vi "psp_supervision.vi"() -> ()   [LabVIEW 2020]
uses:
  archive.ctl
  sync_type_def.ctl
  HT_type-def.ctl
  HF_type_def.ctl
  vacuum_type_def.ctl
  modulator_type_def.ctl
  water_cooling_type_def.ctl
  all_magnets_type_def.ctl
  <resource>/objmgr/ni.var.rc
panel:
  in  "container refnum in":refnum<k21>="ni.var.psp://eureka/SUPERVISION"
  out "archive":T1={"sync"={"elyse/sync/NI6071E/delay"=1.5500000000000005, "elyse/sync/NI6071E/width"=1.0, "elyse/sync/frequency/delay"=10.0, "elyse/sync/frequency/width"=181000.0, "elyse/sync/WCM/delay"=2177.9, "elyse/sync/WCM/width"=10.0, "elyse/sync/modulator/delay"=2182.400000000002, "elyse/sync/modulator/width"=3.0, "elyse/sync/HF/delay"=2175.0, "elyse/sync/HF/width"=3.0, "elyse/sync/Faraday/delay"=5080.0, "elyse/sync/Faraday/width"=100.0, "elyse/sync/Oscilloscope/delay"=2175.0, "elyse/sync/Oscilloscope/width"=2.8, "elyse/sync/50Hz_20MHz/delay"=1.0, "elyse/sync/50Hz_20MHz/width"=5000.0, "elyse/sync/laser_HF/delay"=0.35, "elyse/sync/laser_HF/width"=0.35, "elyse/sync/IMAC/delay"=2176.0, "elyse/sync/IMAC/width"=100.0, "elyse/sync/laser/delay"=2008.3, "elyse/sync/laser/width"=10.0, "elyse/sync/oscilloscope1/delay"=2175.0, "elyse/sync/oscilloscope1/width"=10.0, "elyse/sync/oscilloscope2/delay"=2175.0, "elyse/sync/oscilloscope2/width"=100.0, "elyse/sync/detection1/delay"=500.0, "elyse/sync/detection1/width"=500.0, "elyse/sync/detection1/delay"=0.3, "elyse/sync/detection2/width"=10.0, "elyse/sync/machine/delay"=2175.0, "elyse/sync/machine/width"=100.0, "elyse/sync/n_selection"=4.0}, "HT"={"elyse/HT/voltage/set_value"=6.5, "elyse/HT/voltage/value"=1.5625e-08, "elyse/HT/current/value"=0.0, "elyse/preamplifier/set_value"=1.5625e-08, "elyse/preamplifier/value"=0.0}, "HF"={"elyse/HF/attenuator/value"=-0.01903046052094623, "elyse/HF/dephaser/value"=-18.585806237727724, "elyse/HF/dephaser/value_manuel"=-78.82860725035081, "elyse/HF/canon/value"=0.0, "elyse/HF/section/value"=-18.585806237727724}, "vacuum"={"elyse/vacuum/preparation_chamber/state"=TRUE, "elyse/vacuum/preparation_chamber/measurement"=0.0, "elyse/vacuum/HF/state"=TRUE, "elyse/vacuum/HF/measurement"=0.0, "elyse/vacuum/canon/state"=TRUE, "elyse/vacuum/canon/measurement"=0.0, "elyse/vacuum/section/state"=TRUE, "elyse/vacuum/section/measurement"=0.0, "elyse/vacuum/dipole1/state"=TRUE, "elyse/vacuum/dipole1/measurement"=0.0, "elyse/vacuum/screen1/state"=TRUE, "elyse/vacuum/screen1/measurement"=0.0, "elyse/vacuum/mirror/state"=TRUE, "elyse/vacuum/mirror/measurement"=0.0, "elyse/vacuum/tpg300_section/state"=TRUE, "elyse/vacuum/tpg300_section/measurement"=0.0, "elyse/vacuum/valves/cathode/state"=FALSE, "elyse/vacuum/valves/injection/state"=FALSE}, "modulator"={"elyse/modulator/focale1/current/value"=0.0, "elyse/modulator/focale2/current/value"=0.0, "elyse/modulator/focale3/current/value"=0.0, "elyse/modulator/LAR/voltage/value"=0.0, "elyse/modulator/line_end/current/value"=0.0, "elyse/modulator/thyratron/currents/power/value"=0.0, "elyse/modulator/thyratron_reservoir/current/value"=0.0, "elyse/modulator/paramagnetization/current/value"=0.0, "elyse/modulator/thyratron/voltages/heating/value"=0.0, "elyse/modulator/thyratron/currents/heating/value"=0.0, "elyse/modulator/klystron/currents/power/value"=0.0, "elyse/modulator/klystron/voltages/power/value"=0.0, "elyse/modulator/klystron/currents/heating/value"=0.0, "elyse/modulator/klystron/voltages/heating/value"=0.0}, "cooling"={"elyse/cooling/section/temperature/set_value"=28.0, "elyse/cooling/section/temperature/measurement"=27.96142578125, "elyse/cooling/canon/temperature/set_value"=20.2, "elyse/cooling/canon/temperature/measurement"=26.69921875}, "magnets"={"elyse/magnets/focale/set_value"=0.0, "elyse/magnets/focale/value"=0.0, "elyse/magnets/phase_HF_laser/set_value"=0.0, "elyse/magnets/phase_HF_laser/value"=0.0, "elyse/magnets/dipole1/set_value"=0.0, "elyse/magnets/dipole1/value"=0.0, "elyse/magnets/dipole2/set_value"=0.0, "elyse/magnets/dipole2/value"=0.0, "elyse/magnets/Cor_H1/set_value"=0.0, "elyse/magnets/Cor_H1/value"=0.0, "elyse/magnets/Cor_V1/set_value"=0.0, "elyse/magnets/Cor_V1/value"=0.0, "elyse/magnets/Cor_H2/set_value"=0.0, "elyse/magnets/Cor_H2/value"=0.0, "elyse/magnets/Cor_V2/set_value"=0.0, "elyse/magnets/Cor_V2/value"=0.0, "elyse/magnets/Cor_H3/set_value"=0.0, "elyse/magnets/Cor_H3/value"=0.0, "elyse/magnets/Cor_V3/set_value"=-5.0, "elyse/magnets/Cor_V3/value"=0.0, "elyse/magnets/Cor_H4/set_value"=0.0, "elyse/magnets/Cor_H4/value"=0.0, "elyse/magnets/Cor_V4/set_value"=0.0, "elyse/magnets/Cor_V4/value"=0.0, "elyse/magnets/Cor_H5/set_value"=0.0, "elyse/magnets/Cor_H5/value"=0.0, "elyse/magnets/Cor_V5/set_value"=0.0, "elyse/magnets/Cor_V5/value"=0.0, "elyse/magnets/triplet1-1/set_value"=0.0, "elyse/magnets/triplet1-1/value"=0.0, "elyse/magnets/triplet1-2/set_value"=0.0, "elyse/magnets/triplet1-2/value"=0.0, "elyse/magnets/triplet2-1/set_value"=0.0, "elyse/magnets/triplet2-1/value"=0.0, "elyse/magnets/triplet2-2/set_value"=0.0, "elyse/magnets/triplet2-2/value"=0.0, "elyse/magnets/qudrupole1/set_value"=0.0, "elyse/magnets/qudrupole1/value"=0.0, "elyse/magnets/qudrupole2/set_value"=0.0, "elyse/magnets/qudrupole2/value"=0.0}, "time"={"elyse/timestamp"=0.0}}
  in  "Stop":bool
  out "Refnum SVE":refnum<k21>[](array[refnum])
  out "error out":errorcluster
  in  "tab":enum32{"  Variables"}(tab)
  in  "Onglet VAR PAR":T9(tab)=enum."C6/9 NI6703"
  out "DPS":T10
  out "EPS":T11
  out "DPC":T12
  out "EPC":T13
  out "C1NI6071E":T14 caption="Cluster 3" {"63 ACH63 b100 Libre ?" format="%.3f"; "62 ACH62 b98 Libre ?" format="%.3f"; "61 ACH61 b96 Libre ?" format="%.3f"; "60 ACH60 b94 Libre ?" format="%.3f"; "59 ACH59 b92 Libre ?" format="%.3f"; "58 ACH58 b90 Libre ?" format="%.3f"; "57 ACH57 b88 Libre ?" format="%.3f"; "56 ACH56 b86 Libre ?" format="%.3f"; "55 ACH55 b99 Libre ?" format="%.3f"; "54 ACH54 b97 Libre ?" format="%.3f"; "53 ACH53 b95 Libre ?" format="%.3f"; "52 ACH52 b93 Libre ?" format="%.3f"; "51 ACH51 b91 Libre ?" format="%.3f"; "50 ACH50 b89 Libre ?" format="%.3f"; "49 ACH49 b87 Libre ?" format="%.3f"; "48 ACH48 b85 Réservé" format="%.3f"; "47 ACH47 b84 Réservé" format="%.3f"; "46 ACH46 b82 Réservé" format="%.3f"; "45 ACH45 b80 Mesure phase HF1" format="%.3f"; "44 ACH44 b78 Mesure Atténuateur" format="%.3f"; "43 ACH43 b74 Réservé" format="%.3f"; "42 ACH42 b72 Mes champ Dipôle 2" format="%.3f"; "41 ACH41 b70 Mes H5" format="%.3f"; "40 ACH40 b68 Mes I correcte Dipôle 21 (H4)" format="%.3f"; "39 ACH39 b83 Réservé" format="%.3f"; "38 ACH38 b81 Mesure phase HF2" format="%.3f"; "37 ACH37 b79 Mes position Déphaseur ajust" format="%.3f"; "36 ACH36 b77 Mes position Déphaseur" format="%.3f"; "35 ACH35 b73 Mes champ Dipôle 2" format="%.3f"; "34 ACH34 b71 Mes I Guidage V5" format="%.3f"; "33 ACH33 b69 Mes I Guidage V4" format="%.3f"; "32 ACH32 b67 Mes I Guidage V3" format="%.3f"; "31 ACH31 b66 Mes I correcte Dipôle 1 (H3)" format="%.3f"; "30 ACH30 b64 Mes I Guidage H2" format="%.3f"; "29 ACH29 b62 Mes I Guidage H1" format="%.3f"; "28 ACH28 b60 Mes I Dipôle 1" format="%.3f"; "27 ACH27 b58 Mes I Quadripôle 2" format="%.3f"; "26 ACH26 b56 Réservé" format="%.3f"; "25 ACH25 b54 Mes I Triplet 2-1" format="%.3f"; "24 ACH24 b52 Mes I Triplet 1-2" format="%.3f"; "23 ACH23 b65 Mes I Guidage V2" format="%.3f"; "22 ACH22 b63 Mes I Guidage V1" format="%.3f"; "21 ACH21 b61 Mes I Dipôle 2" format="%.3f"; "20 ACH20 b59 Mes I Solénoïde" format="%.3f"; "19 ACH19 b57 Mes I Quadripôle 1" format="%.3f"; "18 ACH18 b55 Mes I Triplet 2-2" format="%.3f"; "17 ACH17 b53 Réservé" format="%.3f"; "16 ACH16 b51 Mes I Triplet 1-1" format="%.3f"; "15 ACH15 b18 Libre ?" format="%.3f"; "14 ACH14 b16 Libre ?" format="%.3f"; "13 ACH13 b14 Libre ?" format="%.3f"; "12 ACH12 b12 Mes Vide jauge canon" format="%.3f"; "11 ACH11 b10 Mes Vide DIP 1 (PIQ27 + 33)" format="%.3f"; "10 ACH10 b08 Mes Vide Section (PIQ 16)" format="%.3f"; "09 ACH09 b06 Mes Vide SAS guide HF" format="%.3f"; "08 ACH08 b04 Mes température Section" format="%.3f"; "07 ACH07 b17 Libre ?" format="%.3f"; "06 ACH06 b15 Libre ?" format="%.3f"; "05 ACH05 b13 Libre ?" format="%.3f"; "04 ACH04 b11 Mes Vide Ecran 1 (PIQ 53-63)" format="%.3f"; "03 ACH03 b09 Mes Vide Miroir (PIQ 21)" format="%.3f"; "02 ACH02 b07 Mes Vide Canon (PIQ 12)" format="%.3f"; "01 ACH01 b05 Mes Vide Chambre de préparation" format="%.3f"; "00 ACH00 b03 Mes température Canon" format="%.3f"}
  out "C2NI6071E":T15 caption="Cluster 3" {"63 ACH63 b100 Libre ?" format="%.3f"; "62 ACH62 b98 Libre ?" format="%.3f"; "61 ACH61 b96 Libre ?" format="%.3f"; "60 ACH60 b94 Libre ?" format="%.3f"; "59 ACH59 b92 Libre ?" format="%.3f"; "58 ACH58 b90 Libre ?" format="%.3f"; "57 ACH57 b88 Libre ?" format="%.3f"; "56 ACH56 b86 Signal laser 1" format="%.3f"; "55 ACH55 b99 Libre ?" format="%.3f"; "54 ACH54 b97 Libre ?" format="%.3f"; "53 ACH53 b95 Libre ?" format="%.3f"; "52 ACH52 b93 Libre ?" format="%.3f"; "51 ACH51 b91 Libre ?" format="%.3f"; "50 ACH50 b89 Libre ?" format="%.3f"; "49 ACH49 b87 Signal laser 2" format="%.3f"; "48 ACH48 b85 Mes position Miroir Y" format="%.3f"; "47 ACH47 b84 Mes position Miroir X" format="%.3f"; "46 ACH46 b82 Mes I obcs Faraday 3" format="%.3f"; "45 ACH45 b80 Mes I obcs Faraday 1" format="%.3f"; "44 ACH44 b78 Mes position Ecran 2" format="%.3f"; "43 ACH43 b74 Mes Fente V position mors B" format="%.3f"; "42 ACH42 b72 Mes Fente H position mors G" format="%.3f"; "41 ACH41 b70 Mes WCM 5" format="%.3f"; "40 ACH40 b68 Mes WCM 3" format="%.3f"; "39 ACH39 b83 Libre ?" format="%.3f"; "38 ACH38 b81 Mes I obcs Faraday 2" format="%.3f"; "37 ACH37 b79 Mes position Ecran 3" format="%.3f"; "36 ACH36 b77 Mes position Ecran 1" format="%.3f"; "35 ACH35 b73 Mes Fente V position mors H" format="%.3f"; "34 ACH34 b71 Mes Fente H position mors D" format="%.3f"; "33 ACH33 b69 Mes WCM 4" format="%.3f"; "32 ACH32 b67 Mes WCM 2D" format="%.3f"; "31 ACH31 b66 Mes WCM 2G" format="%.3f"; "30 ACH30 b64 Mes WCM 2H" format="%.3f"; "29 ACH29 b62 Mes WCM 1G" format="%.3f"; "28 ACH28 b60 Mes WCM 1H" format="%.3f"; "27 ACH27 b58 Mes I Faraday 2" format="%.3f"; "26 ACH26 b56 Mes HF directe Section" format="%.3f"; "25 ACH25 b54 Réservé" format="%.3f"; "24 ACH24 b52 Mes I Klystron" format="%.3f"; "23 ACH23 b65 Mes WCM 2B" format="%.3f"; "22 ACH22 b63 Mes WCM 1D" format="%.3f"; "21 ACH21 b61 Mes WCM 1B" format="%.3f"; "20 ACH20 b59 Mes I Faraday 3" format="%.3f"; "19 ACH19 b57 Mes I Faraday 1" format="%.3f"; "18 ACH18 b55 Mes HF directe Canon" format="%.3f"; "17 ACH17 b53 Mes V LAR" format="%.3f"; "16 ACH16 b51 Mes V Klystron" format="%.3f"; "15 ACH15 b18 Mes I alimentation HT" format="%.3f"; "14 ACH14 b16 Libre ?" format="%.3f"; "13 ACH13 b14 Mes I Focalisateur 2" format="%.3f"; "12 ACH12 b12 Mes I fin de Ligne" format="%.3f"; "11 ACH11 b10 Mes I Thyratron" format="%.3f"; "10 ACH10 b08 Mes I Réservoir Thyratron" format="%.3f"; "09 ACH09 b06 Mes I  Chauffage Klystron" format="%.3f"; "08 ACH08 b04 Mes I Chauffage Thyratron" format="%.3f"; "07 ACH07 b17 Mes V alimentation HT" format="%.3f"; "06 ACH06 b15 Mes I Focalisateur 3" format="%.3f"; "05 ACH05 b13 Mes I Focalisateur 1" format="%.3f"; "04 ACH04 b11 Mes I Prémagnétisation" format="%.3f"; "03 ACH03 b09 Réservé" format="%.3f"; "02 ACH02 b07 Mes I D'Qing" format="%.3f"; "01 ACH01 b05 Mes V Chauffage Klystron" format="%.3f"; "00 ACH00 b03 Mes V Chauffage Thyratron" format="%.3f"}
  out "C3_IN_DIO96":T16 caption="Cluster 3"
  out "C3_OUT_DIO96":T17 caption="Cluster 3"
  out "C4_IN_DIO96":T18 caption="Cluster 3"
  out "C4_OUT_DIO96":T19 caption="Cluster 3"
  out "C5_IN_DIO96":T20 caption="Cluster 3"
  out "C5_OUT_DIO96":T21 caption="Cluster 3"
  out "C6NI6703":T22 caption="Cluster 3" {"09 OUT09 b37 Cmd Guidage V5" format="%.3f"; "08 OUT08 b33 Réserve" format="%.3f"; "07 OUT07 b29 Cmd Guidage V4" format="%.3f"; "06 OUT06 b25 Cmd Guidage H4" format="%.3f"; "05 OUT05 b21 Cmd Guidage V3" format="%.3f"; "04 OUT04 b17 Cmd Guidage H3" format="%.3f"; "03 OUT03 b13 Cmd Guidage V2" format="%.3f"; "02 OUT02 b09 Cmd Guidage H2" format="%.3f"; "01 OUT01 b05 Cmd Guidage V1" format="%.3f"; "00 OUT00 b01 Cmd Guidage H1" format="%.3f"}
  out "C7NI6703":T23 caption="Cluster 3" {"09 OUT09 b37 Cmd I Dipôle 2" format="%.3f"; "08 OUT08 b33 Cmd I Dipôle 1" format="%.3f"; "07 OUT07 b29 Cmd I Quad 2" format="%.3f"; "06 OUT06 b25 Cmd I Quad 1" format="%.3f"; "05 OUT05 b21 Cmd I Solénoïde" format="%.3f"; "04 OUT04 b17 Cmd I Triplet 2-2" format="%.3f"; "03 OUT03 b13 Cmd I Triplet 2-1" format="%.3f"; "02 OUT02 b09 Réserve" format="%.3f"; "01 OUT01 b05 Cmd I Triplet 1-2" format="%.3f"; "00 OUT00 b01 Cmd I Triplet 1-1" format="%.3f"}
  out "C8NI6703":T24 caption="Cluster 3" {"09 OUT09 b37 Cmd position Miroir Y" format="%.3f"; "08 OUT08 b33 Cmd position Miroir X" format="%.3f"; "07 OUT07 b29 Réserve" format="%.3f"; "06 OUT06 b25 Cmd amplitude HF préampli" format="%.3f"; "05 OUT05 b21 Cmd déphasage HF/LASER" format="%.3f"; "04 OUT04 b17 Cmd Pos. Atténuateur" format="%.3f"; "03 OUT03 b13 Cmd Pos. Déphaseur" format="%.3f"; "02 OUT02 b09 Cmd Temp. Section" format="%.3f"; "01 OUT01 b05 Cmd Temp. Canon" format="%.3f"; "00 OUT00 b01 Réserve" format="%.3f"}
  out "C9NI6703":T25 caption="Cluster 3" {"09 OUT09 b37 Réserve" format="%.3f"; "08 OUT08 b33 Réserve" format="%.3f"; "07 OUT07 b29 Réserve" format="%.3f"; "06 OUT06 b25 Cmd position translateur Ecran 3" format="%.3f"; "05 OUT05 b21 Cmd position translateur Ecran 2" format="%.3f"; "04 OUT04 b17 Cmd position translateur Ecran 1" format="%.3f"; "03 OUT03 b13 Cmd position fente HD" format="%.3f"; "02 OUT02 b09 Cmd position fente HG" format="%.3f"; "01 OUT01 b05 Cmd DeQing" format="%.3f"; "00 OUT00 b01 Cmd alimentation HT" format="%.3f"}
  out "C1011NI6602":T26 caption="Cluster 3" {"N° du compteur" format="%.3f"; "31 OUT07 b16 C11 Largeur" format="%.3f"; "30 OUT07 b16 C11 Délais" format="%.3f"; "29 OUT06 b53 C11 Largeur" format="%.3f"; "28 OUT06 b53 C11 Délais" format="%.3f"; "27 OUT05 b23 C11 Largeur" format="%.3f"; "26 OUT05 b23 C11 Délais" format="%.3f"; "25 OUT04 b26 C11 Largeur" format="%.3f"; "24 OUT04 b26 C11 Délais" format="%.3f"; "23 OUT03 b29 C11 Largeur" format="%.3f"; "22 OUT03 b29 C11 Délais" format="%.3f"; "21 OUT02 b32 C11 Largeur" format="%.3f"; "20 OUT02 b32 C11 Délais" format="%.3f"; "19 OUT01 b09 C11 Largeur" format="%.3f"; "18 OUT01 b09 C11 Délais" format="%.3f"; "17 OUT00 b05 C11 Largeur" format="%.3f"; "16 OUT00 b05 C11 Délais" format="%.3f"; "15 OUT07 b16 C10 Largeur" format="%.3f"; "14 OUT07 b16 C10 Délais" format="%.3f"; "13 OUT06 b53 C10 Largeur" format="%.3f"; "12 OUT06 b53 C10 Délais" format="%.3f"; "11 OUT05 b23 C10 Largeur" format="%.3f"; "10 OUT05 b23 C10 Délais" format="%.3f"; "09 OUT04 b26 C10 Largeur" format="%.3f"; "08 OUT04 b26 C10 Délais" format="%.3f"; "07 OUT03 b29 C10 Largeur" format="%.3f"; "06 OUT03 b29 C10 Délais" format="%.3f"; "05 OUT02 b32 C10 Largeur" format="%.3f"; "04 OUT02 b32 C10 Délais" format="%.3f"; "03 OUT01 b09 C10 Largeur" format="%.3f"; "02 OUT01 b09 C10 Délais" format="%.3f"; "01 OUT00 b05 C10 Largeur" format="%.3f"; "00 OUT00 b05 C10 Délais" format="%.3f"}
  out "C12NI1409":string
  out "VDM-S":T27 caption="Cluster 3"
  out "VDM-A":T28 caption="Cluster 3"
  out "VDD":T27 caption="Cluster 3"
  out "VAM-S":T29 caption="Cluster 3" {"63" format="%.4g"; "62" format="%.4g"; "61" format="%.4g"; "60" format="%.4g"; "59" format="%.4g"; "58" format="%.4g"; "57" format="%.4g"; "56" format="%.4g"; "55" format="%.4g"; "54" format="%.4g"; "53" format="%.4g"; "52" format="%.4g"; "51" format="%.4g"; "50" format="%.4g"; "49" format="%.4g"; "48" format="%.4g"; "47" format="%.4g"; "46" format="%.4g"; "45" format="%.4g"; "44" format="%.4g"; "43" format="%.4g"; "42" format="%.4g"; "41" format="%.4g"; "40" format="%.4g"; "39" format="%.4g"; "38" format="%.4g"; "37" format="%.4g"; "36" format="%.4g"; "35" format="%.4g"; "34" format="%.4g"; "33" format="%.4g"; "32" format="%.4g"; "31" format="%.4g"; "30" format="%.4g"; "29" format="%.4g"; "28" format="%.4g"; "27" format="%.4g"; "26" format="%.4g"; "25" format="%.4g"; "24" format="%.4g"; "23" format="%.4g"; "22" format="%.4g"; "21" format="%.4g"; "20" format="%.4g"; "19" format="%.4g"; "18" format="%.4g"; "17" format="%.4g"; "16" format="%.4g"; "15" format="%.4g"; "14" format="%.4g"; "13" format="%.4g"; "12" format="%.4g"; "11" format="%.4g"; "10" format="%.4g"; "09" format="%.4g"; "08" format="%.4g"; "07" format="%.4g"; "06" format="%.4g"; "05" format="%.4g"; "04" format="%.4g"; "03" format="%.4g"; "02 SUP Evenement" format="%.4g"; "01 SUP Variables" format="%.4g"; "00 SUP Vidéo" format="%.4g"}
  out "VAM-A":T30 caption="Cluster 3" {"63 B_NI6220" format="%.4g"; "62" format="%.4g"; "61" format="%.4g"; "60" format="%.4g"; "59" format="%.4g"; "58" format="%.4g"; "57" format="%.4g"; "56" format="%.4g"; "55" format="%.4g"; "54" format="%.4g"; "53" format="%.4g"; "52" format="%.4g"; "51" format="%.4g"; "50" format="%.4g"; "49" format="%.4g"; "48" format="%.4g"; "47" format="%.4g"; "46" format="%.4g"; "45" format="%.4g"; "44" format="%.4g"; "43" format="%.4g"; "42" format="%.4g"; "41" format="%.4g"; "40" format="%.4g"; "39 WCM2DMin" format="%.4g"; "38 WCM2GMin" format="%.4g"; "37 WCM2BMin" format="%.4g"; "36 WCM2HMin" format="%.4g"; "35 WCM2DMax" format="%.4g"; "34 WCM2GMax" format="%.4g"; "33 WCM2BMax" format="%.4g"; "32 WCM2HMax" format="%.4g"; "31" format="%.4g"; "30" format="%.4g"; "29" format="%.4g"; "28" format="%.4g"; "27" format="%.4g"; "26" format="%.4g"; "25" format="%.4g"; "24" format="%.4g"; "23" format="%.4g"; "22" format="%.4g"; "21" format="%.4g"; "20 ACQ Vide TPG300 PIQ63" format="%.4g"; "19 ACQ Libre" format="%.5g"; "18 ACQ Libre" format="%.5g"; "17 ACQ Vide Ecran PIQ53/63" format="%.5g"; "16 ACQ Vide Dip PIQ27/33" format="%.5g"; "15 ACQ Vide Miroir PIQ21" format="%.5g"; "14 ACQ Vide Section PIQ16" format="%.5g"; "13 ACQ Vide Canon PIQ12" format="%.5g"; "12 ACQ Vide PI Guide HF" format="%.5f"; "11 ACQ Vide Chambre" format="%.4g"; "10 ACQ Vide Section" format="%.4g"; "09" format="%.4g"; "08" format="%.4g"; "07" format="%.4g"; "06" format="%.4g"; "05" format="%.4g"; "04" format="%.4g"; "03" format="%.4g"; "02 ACQ Evénement" format="%.4g"; "01 ACQ Variables" format="%.4g"; "00 ACQ Auxiliare" format="%.4g"}
  out "VAD":T31 caption="Cluster 3" {"63" format="%.4g"; "62" format="%.4g"; "61" format="%.4g"; "60" format="%.4g"; "59" format="%.4g"; "58" format="%.4g"; "57" format="%.4g"; "56" format="%.4g"; "55" format="%.4g"; "54" format="%.4g"; "53" format="%.4g"; "52" format="%.4g"; "51" format="%.4g"; "50" format="%.4g"; "49" format="%.4g"; "48" format="%.4g"; "47" format="%.4g"; "46" format="%.4g"; "45" format="%.4g"; "44" format="%.4g"; "43" format="%.4g"; "42" format="%.4g"; "41" format="%.4g"; "40" format="%.4g"; "39" format="%.4g"; "38" format="%.4g"; "37" format="%.4g"; "36" format="%.4g"; "35" format="%.4g"; "34" format="%.4g"; "33" format="%.4g"; "32" format="%.4g"; "31" format="%.4g"; "30" format="%.4g"; "29" format="%.4g"; "28" format="%.4g"; "27" format="%.4g"; "26" format="%.4g"; "25" format="%.4g"; "24" format="%.4g"; "23" format="%.4g"; "22" format="%.4g"; "21" format="%.4g"; "20" format="%.4g"; "19" format="%.4g"; "18" format="%.4g"; "17" format="%.4g"; "16" format="%.4g"; "15" format="%.4g"; "14" format="%.4g"; "13" format="%.4g"; "12" format="%.4g"; "11" format="%.4g"; "10" format="%.4g"; "09" format="%.4g"; "08" format="%.4g"; "07" format="%.4g"; "06" format="%.4g"; "05" format="%.4g"; "04" format="%.4g"; "03" format="%.4g"; "02" format="%.4g"; "01" format="%.4g"; "00" format="%.4g"}
  out "VTL":string[](array[string])
  out "VTS":string[](array[string])
  out "VTA":string[](array[string])
  # "Légende:\n\nLes Procédure simples sont des actions uniques sur un éléments ou groupe d'éléments.\nSelon les élements mis en oeuvre l'état OK de fin de procédure dépend de la remontée ou non de paramêtres de contrôle.\n\nLes Procédures combinées mettent en oeuvre une suites de procédures simples et correspondent à un état précis d'Elyse:\n(TIR - PRETIR-VEILLE - ARRET)\n\nSDC: Salle De Contrôle.\nX: Correspond à une demande de l'utilisateur depuis la SDC ou d'un pilotage distant.\nED: En Défaut.\nI: Etats transitoire (ex: entre TIR et Veille).\n1 2 3 4: correspond aux étapes intermédiaires de démarrage du modulateur.\nReset: Signifie une remise à zéro des défauts ce qui permet de passer à l'étape suivante.\nOK: Correspond à un une fin de procédure normale sans défaut.\nX EC: Correspond à un flag indiquant une demande de procédure combinée en cours.\nDPS: Cluster de Demande de Prcédure Simples (Read PC-ACQ / Write PC-SUP)\nEPS: Cluster d'Etats des Procédures Simples (Write PC-ACQ / Read PC-SUP)\nDPC: Cluster de Demande de Procédure Combinées (Read PC-ACQ / Write PC-SUP)\nEPC: Cluster d'états des Procédures Combinées (Write PC-ACQ / Read PC-SUP)"
  # "Cluster d'entrée des 64 voies analogiques de la carte C1 PCI 6071E"
  # "Cluster d'entrée des 64 voies analogiques de la carte C2 PCI 6071E"
  # "Cluster d'entrée des 56 voies numériques de la carte C3 DIO96"
  # "Cluster de sortie des 40 voies \nnumériques de la carte C3 DIO96"
  # "Cluster d'entrée des 64 voies numériques de la carte C4 DIO96"
  # "Cluster de sortie des 32 voies numériques \nde la carte C4 DIO96"
  # "Cluster d'entrée des 56 voies numériques de la carte C5 DIO96"
  # "Cluster de sortie des 40 voies numériques\nde la carte C5 DIO96"
  # "Cluster de sortie des 9 voies analogiques des 4 cartes C6,C7,C8,C9 PCI6703"
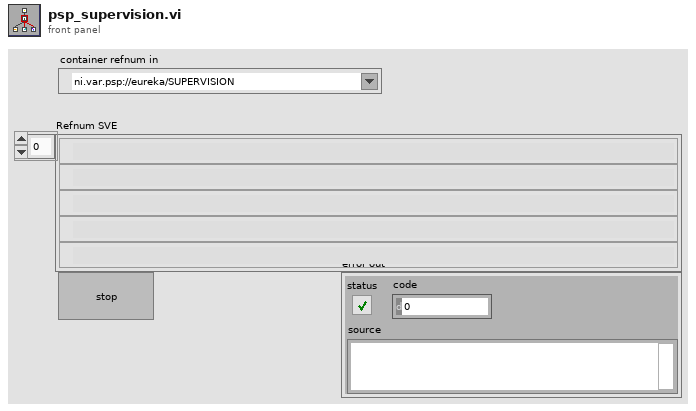
[diagram p1: front panel]
types:
  T1 = typedef "archive.ctl" = cluster{"sync":T2, "HT":T3, "HF":T4, "vacuum":T5, "modulator":T6, "cooling":T7, "magnets":T8, "time":cluster{"elyse/timestamp":dbl}}
  T2 = typedef "sync_type_def.ctl" = cluster{"elyse/sync/NI6071E/delay":dbl, "elyse/sync/NI6071E/width":dbl, "elyse/sync/frequency/delay":dbl, "elyse/sync/frequency/width":dbl, "elyse/sync/WCM/delay":dbl, "elyse/sync/WCM/width":dbl, "elyse/sync/modulator/delay":dbl, "elyse/sync/modulator/width":dbl, "elyse/sync/HF/delay":dbl, "elyse/sync/HF/width":dbl, "elyse/sync/Faraday/delay":dbl, "elyse/sync/Faraday/width":dbl, "elyse/sync/Oscilloscope/delay":dbl, "elyse/sync/Oscilloscope/width":dbl, "elyse/sync/50Hz_20MHz/delay":dbl, "elyse/sync/50Hz_20MHz/width":dbl, "elyse/sync/laser_HF/delay":dbl, "elyse/sync/laser_HF/width":dbl, "elyse/sync/IMAC/delay":dbl, "elyse/sync/IMAC/width":dbl, "elyse/sync/laser/delay":dbl, "elyse/sync/laser/width":dbl, "elyse/sync/oscilloscope1/delay":dbl, "elyse/sync/oscilloscope1/width":dbl, "elyse/sync/oscilloscope2/delay":dbl, "elyse/sync/oscilloscope2/width":dbl, "elyse/sync/detection1/delay":dbl, "elyse/sync/detection1/width":dbl, "elyse/sync/detection1/delay":dbl, "elyse/sync/detection2/width":dbl, "elyse/sync/machine/delay":dbl, "elyse/sync/machine/width":dbl, "elyse/sync/n_selection":dbl}
  T3 = typedef "HT_type-def.ctl" = cluster{"elyse/HT/voltage/set_value":dbl, "elyse/HT/voltage/value":dbl, "elyse/HT/current/value":dbl, "elyse/preamplifier/set_value":dbl, "elyse/preamplifier/value":dbl}
  T4 = typedef "HF_type_def.ctl" = cluster{"elyse/HF/attenuator/value":dbl, "elyse/HF/dephaser/value":dbl, "elyse/HF/dephaser/value_manuel":dbl, "elyse/HF/canon/value":dbl, "elyse/HF/section/value":dbl}
  T5 = typedef "vacuum_type_def.ctl" = cluster{"elyse/vacuum/preparation_chamber/state":bool, "elyse/vacuum/preparation_chamber/measurement":dbl, "elyse/vacuum/HF/state":bool, "elyse/vacuum/HF/measurement":dbl, "elyse/vacuum/canon/state":bool, "elyse/vacuum/canon/measurement":dbl, "elyse/vacuum/section/state":bool, "elyse/vacuum/section/measurement":dbl, "elyse/vacuum/dipole1/state":bool, "elyse/vacuum/dipole1/measurement":dbl, "elyse/vacuum/screen1/state":bool, "elyse/vacuum/screen1/measurement":dbl, "elyse/vacuum/mirror/state":bool, "elyse/vacuum/mirror/measurement":dbl, "elyse/vacuum/tpg300_section/state":bool, "elyse/vacuum/tpg300_section/measurement":dbl, "elyse/vacuum/valves/cathode/state":bool, "elyse/vacuum/valves/injection/state":bool}
  T6 = typedef "modulator_type_def.ctl" = cluster{"elyse/modulator/focale1/current/value":dbl, "elyse/modulator/focale2/current/value":dbl, "elyse/modulator/focale3/current/value":dbl, "elyse/modulator/LAR/voltage/value":dbl, "elyse/modulator/line_end/current/value":dbl, "elyse/modulator/thyratron/currents/power/value":dbl, "elyse/modulator/thyratron_reservoir/current/value":dbl, "elyse/modulator/paramagnetization/current/value":dbl, "elyse/modulator/thyratron/voltages/heating/value":dbl, "elyse/modulator/thyratron/currents/heating/value":dbl, "elyse/modulator/klystron/currents/power/value":dbl, "elyse/modulator/klystron/voltages/power/value":dbl, "elyse/modulator/klystron/currents/heating/value":dbl, "elyse/modulator/klystron/voltages/heating/value":dbl}
  T7 = typedef "water_cooling_type_def.ctl" = cluster{"elyse/cooling/section/temperature/set_value":dbl, "elyse/cooling/section/temperature/measurement":dbl, "elyse/cooling/canon/temperature/set_value":dbl, "elyse/cooling/canon/temperature/measurement":dbl}
  T8 = typedef "all_magnets_type_def.ctl" = cluster{"elyse/magnets/focale/set_value":dbl, "elyse/magnets/focale/value":dbl, "elyse/magnets/phase_HF_laser/set_value":dbl, "elyse/magnets/phase_HF_laser/value":dbl, "elyse/magnets/dipole1/set_value":dbl, "elyse/magnets/dipole1/value":dbl, "elyse/magnets/dipole2/set_value":dbl, "elyse/magnets/dipole2/value":dbl, "elyse/magnets/Cor_H1/set_value":dbl, "elyse/magnets/Cor_H1/value":dbl, "elyse/magnets/Cor_V1/set_value":dbl, "elyse/magnets/Cor_V1/value":dbl, "elyse/magnets/Cor_H2/set_value":dbl, "elyse/magnets/Cor_H2/value":dbl, "elyse/magnets/Cor_V2/set_value":dbl, "elyse/magnets/Cor_V2/value":dbl, "elyse/magnets/Cor_H3/set_value":dbl, "elyse/magnets/Cor_H3/value":dbl, "elyse/magnets/Cor_V3/set_value":dbl, "elyse/magnets/Cor_V3/value":dbl, "elyse/magnets/Cor_H4/set_value":dbl, "elyse/magnets/Cor_H4/value":dbl, "elyse/magnets/Cor_V4/set_value":dbl, "elyse/magnets/Cor_V4/value":dbl, "elyse/magnets/Cor_H5/set_value":dbl, "elyse/magnets/Cor_H5/value":dbl, "elyse/magnets/Cor_V5/set_value":dbl, "elyse/magnets/Cor_V5/value":dbl, "elyse/magnets/triplet1-1/set_value":dbl, "elyse/magnets/triplet1-1/value":dbl, "elyse/magnets/triplet1-2/set_value":dbl, "elyse/magnets/triplet1-2/value":dbl, "elyse/magnets/triplet2-1/set_value":dbl, "elyse/magnets/triplet2-1/value":dbl, "elyse/magnets/triplet2-2/set_value":dbl, "elyse/magnets/triplet2-2/value":dbl, "elyse/magnets/qudrupole1/set_value":dbl, "elyse/magnets/qudrupole1/value":dbl, "elyse/magnets/qudrupole2/set_value":dbl, "elyse/magnets/qudrupole2/value":dbl}
  T9 = enum32{"DPS/C   EPS/C", "C1 NI6071E", "C2 NI6071E", "C3 DIO96 IN", "C3 DIO96 OUT", "C4 DIO96 IN", "C4 DIO96 OUT", "C5 DIO96 IN", "C5 DIO96 OUT", "C6/9 NI6703", "C10-11 NI6602", "C12 NI1409", "VDM-A/S", "VDD", "VAM-A/S", "VAD", "VTA/S/L"}
  T10 = cluster{"Marche refroidissement X":bool, "Arret refroidissement X":bool, " X Marche GENERAL Mod.":bool, "X Arrêt GENERAL Mod.":bool, "X Marche CHAUFFAGE Mod.":bool, "X Arrêt CHAUFFAGE Mod.":bool, "X Marche PREMA Mod. ":bool, "X Arrêt PREMA Mod.":bool, " X Marche RELAIS HT Mod.":bool, "X Arrêt RELAIS HT Mod.":bool, "X Marche FOCALE Mod.":bool, "X Arrêt FOCALE Mod.":bool, "X RESET Mod.":bool, "X Marche Att Déph":bool, "X Arret Att Déph":bool, "X Marche alimentation HT":bool, "X Reset alimentation HT":bool, "X Arrêt alimentation HT":bool, "X Marche impulsion mod":bool, "X Arret impulsion mod":bool, "X Marche alimentation aimant":bool, "X Alimentation aimant = 0V":bool, "X Alimentation aimant = PT":bool, "X Arrêt alimentation aimant":bool, "X Tempo 1s":bool, "X Tempo 5s":bool, "X Tempo 30s":bool, "X FREQ. ELYSE":bool, "Libre X":bool}
  T11 = cluster{"Marche refroidissement":bool, "Marche refroidissement ED":bool, "Marche refroidissement OK":bool, "Arrêt refroidissement":bool, "Arret refroidissement ED":bool, "Arret refroidissement OK":bool, "Marche GENERAL Mod.":bool, "Marche GENERAL Mod. ED":bool, "Marche GENERAL Mod. OK":bool, "Arrêt GENERAL Mod.":bool, "Arrêt GENERAL Mod. ED":bool, "Arrêt GENERAL Mod. OK":bool, "Marche CHAUFFAGE Mod.":bool, "Marche CHAUFFAGE Mod. ED":bool, "Marche CHAUFFAGE Mod. OK":bool, "Arrêt CHAUFFAGE Mod.":bool, "Arrêt CHAUFFAGE Mod. ED":bool, "Arrêt CHAUFFAGE Mod. OK":bool, "Marche PREMA Mod.":bool, "Marche PREMA Mod. ED":bool, "Marche PREMA Mod. OK":bool, "Arrêt PREMA Mod.":bool, "Arrêt PREMA Mod. ED":bool, "Arrêt PREMA Mod. OK":bool, "Marche RELAIS HT Mod.":bool, "Marche RELAIS HT Mod. ED":bool, "Marche RELAIS HT Mod. OK":bool, "Arrêt RELAIS HT Mod.":bool, "Arrêt RELAIS HT Mod. ED":bool, "Arrêt RELAIS HT Mod. OK":bool, "Marche FOCALE Mod.":bool, "Marche FOCALE Mod. ED":bool, "Marche FOCALE Mod. OK":bool, "Arrêt FOCALE Mod.":bool, "Arrêt FOCALE Mod. ED":bool, "Arrêt FOCALE Mod. OK":bool, "RESET Mod.":bool, "Marche Att et Déph HF":bool, "Marche Att Déph ED":bool, "Marche Att Déph OK":bool, "Arrêt Att et Déph HF":bool, "Arret Att Déph ED":bool, "Arret Att Déph OK":bool, "Marche alimentation HT":bool, "Marche alimentation HT ED":bool, "Marche alimentation HT OK":bool, "Reset alimentation HT":bool, "Arrêt alimentation HT":bool, "Arret alimentation HT ED":bool, "Arret alimentation HT OK":bool, "Marche impulsion modulateur":bool, "Marche impulsion mod ED":bool, "Marche impulsion mod OK":bool, "Arrêt impulsion modulateur":bool, "Arret impulsion mod ED":bool, "Arret impulsion mod OK":bool, "Marche alimentation aimants":bool, "Marche alimentation aimant ED":bool, "Marche alimentation aimant OK":bool, "Alimentation aimant = 0V":bool, "Alimentation aimant = 0V ED":bool, "Alimentation aimant = 0V OK":bool, "Alimentation aimant = PT":bool, "Alimentation aimant = PT ED":bool, "Alimentation aimant = PT OK":bool, "Arrêt alimentation aimants":bool, "Arret alimentation aimant ED":bool, "Arret alimentation aimant OK":bool, "Tempo 1s":bool, "Tempo 5s":bool, "Tempo 30s":bool, "FREQ. ELYSE":bool, "FREQ. ELYSE ED":bool, "FREQ. ELYSE OK":bool, "Libre":bool, "Libre ED":bool, "Libre OK":bool}
  T12 = cluster{"TIR X":bool, "PRETIR X":bool, "VEILLE X":bool, "ARRET X":bool, "QUIT X":bool}
  T13 = cluster{"TIR OK":bool, "PRETIR OK":bool, "VEILLE OK":bool, "ARRET OK":bool, "ARRET <> VEILLE":bool, "TIR ED":bool, "PRETIR ED":bool, "VEILLE ED":bool, "VEILLE ED 2":bool, "PRETIR <> VEILLE":bool, "TIR <> PRETIR":bool, "Procédure combiné EC":bool}
  T14 = cluster{"00 ACH00 b03 Mes température Canon":dbl, "01 ACH01 b05 Mes Vide Chambre de préparation":dbl, "02 ACH02 b07 Mes Vide Canon (PIQ 12)":dbl, "03 ACH03 b09 Mes Vide Miroir (PIQ 21)":dbl, "04 ACH04 b11 Mes Vide Ecran 1 (PIQ 53-63)":dbl, "05 ACH05 b13 Libre ?":dbl, "06 ACH06 b15 Libre ?":dbl, "07 ACH07 b17 Libre ?":dbl, "08 ACH08 b04 Mes température Section":dbl, "09 ACH09 b06 Mes Vide SAS guide HF":dbl, "10 ACH10 b08 Mes Vide Section (PIQ 16)":dbl, "11 ACH11 b10 Mes Vide DIP 1 (PIQ27 + 33)":dbl, "12 ACH12 b12 Mes Vide jauge canon":dbl, "13 ACH13 b14 Libre ?":dbl, "14 ACH14 b16 Libre ?":dbl, "15 ACH15 b18 Libre ?":dbl, "16 ACH16 b51 Mes I Triplet 1-1":dbl, "17 ACH17 b53 Réservé":dbl, "18 ACH18 b55 Mes I Triplet 2-2":dbl, "19 ACH19 b57 Mes I Quadripôle 1":dbl, "20 ACH20 b59 Mes I Solénoïde":dbl, "21 ACH21 b61 Mes I Dipôle 2":dbl, "22 ACH22 b63 Mes I Guidage V1":dbl, "23 ACH23 b65 Mes I Guidage V2":dbl, "24 ACH24 b52 Mes I Triplet 1-2":dbl, "25 ACH25 b54 Mes I Triplet 2-1":dbl, "26 ACH26 b56 Réservé":dbl, "27 ACH27 b58 Mes I Quadripôle 2":dbl, "28 ACH28 b60 Mes I Dipôle 1":dbl, "29 ACH29 b62 Mes I Guidage H1":dbl, "30 ACH30 b64 Mes I Guidage H2":dbl, "31 ACH31 b66 Mes I correcte Dipôle 1 (H3)":dbl, "32 ACH32 b67 Mes I Guidage V3":dbl, "33 ACH33 b69 Mes I Guidage V4":dbl, "34 ACH34 b71 Mes I Guidage V5":dbl, "35 ACH35 b73 Mes champ Dipôle 2":dbl, "36 ACH36 b77 Mes position Déphaseur":dbl, "37 ACH37 b79 Mes position Déphaseur ajust":dbl, "38 ACH38 b81 Mesure phase HF2":dbl, "39 ACH39 b83 Réservé":dbl, "40 ACH40 b68 Mes I correcte Dipôle 21 (H4)":dbl, "41 ACH41 b70 Mes H5":dbl, "42 ACH42 b72 Mes champ Dipôle 2":dbl, "43 ACH43 b74 Réservé":dbl, "44 ACH44 b78 Mesure Atténuateur":dbl, "45 ACH45 b80 Mesure phase HF1":dbl, "46 ACH46 b82 Réservé":dbl, "47 ACH47 b84 Réservé":dbl, "48 ACH48 b85 Réservé":dbl, "49 ACH49 b87 Libre ?":dbl, "50 ACH50 b89 Libre ?":dbl, "51 ACH51 b91 Libre ?":dbl, "52 ACH52 b93 Libre ?":dbl, "53 ACH53 b95 Libre ?":dbl, "54 ACH54 b97 Libre ?":dbl, "55 ACH55 b99 Libre ?":dbl, "56 ACH56 b86 Libre ?":dbl, "57 ACH57 b88 Libre ?":dbl, "58 ACH58 b90 Libre ?":dbl, "59 ACH59 b92 Libre ?":dbl, "60 ACH60 b94 Libre ?":dbl, "61 ACH61 b96 Libre ?":dbl, "62 ACH62 b98 Libre ?":dbl, "63 ACH63 b100 Libre ?":dbl}
  T15 = cluster{"00 ACH00 b03 Mes V Chauffage Thyratron":dbl, "01 ACH01 b05 Mes V Chauffage Klystron":dbl, "02 ACH02 b07 Mes I D'Qing":dbl, "03 ACH03 b09 Réservé":dbl, "04 ACH04 b11 Mes I Prémagnétisation":dbl, "05 ACH05 b13 Mes I Focalisateur 1":dbl, "06 ACH06 b15 Mes I Focalisateur 3":dbl, "07 ACH07 b17 Mes V alimentation HT":dbl, "08 ACH08 b04 Mes I Chauffage Thyratron":dbl, "09 ACH09 b06 Mes I  Chauffage Klystron":dbl, "10 ACH10 b08 Mes I Réservoir Thyratron":dbl, "11 ACH11 b10 Mes I Thyratron":dbl, "12 ACH12 b12 Mes I fin de Ligne":dbl, "13 ACH13 b14 Mes I Focalisateur 2":dbl, "14 ACH14 b16 Libre ?":dbl, "15 ACH15 b18 Mes I alimentation HT":dbl, "16 ACH16 b51 Mes V Klystron":dbl, "17 ACH17 b53 Mes V LAR":dbl, "18 ACH18 b55 Mes HF directe Canon":dbl, "19 ACH19 b57 Mes I Faraday 1":dbl, "20 ACH20 b59 Mes I Faraday 3":dbl, "21 ACH21 b61 Mes WCM 1B":dbl, "22 ACH22 b63 Mes WCM 1D":dbl, "23 ACH23 b65 Mes WCM 2B":dbl, "24 ACH24 b52 Mes I Klystron":dbl, "25 ACH25 b54 Réservé":dbl, "26 ACH26 b56 Mes HF directe Section":dbl, "27 ACH27 b58 Mes I Faraday 2":dbl, "28 ACH28 b60 Mes WCM 1H":dbl, "29 ACH29 b62 Mes WCM 1G":dbl, "30 ACH30 b64 Mes WCM 2H":dbl, "31 ACH31 b66 Mes WCM 2G":dbl, "32 ACH32 b67 Mes WCM 2D":dbl, "33 ACH33 b69 Mes WCM 4":dbl, "34 ACH34 b71 Mes Fente H position mors D":dbl, "35 ACH35 b73 Mes Fente V position mors H":dbl, "36 ACH36 b77 Mes position Ecran 1":dbl, "37 ACH37 b79 Mes position Ecran 3":dbl, "38 ACH38 b81 Mes I obcs Faraday 2":dbl, "39 ACH39 b83 Libre ?":dbl, "40 ACH40 b68 Mes WCM 3":dbl, "41 ACH41 b70 Mes WCM 5":dbl, "42 ACH42 b72 Mes Fente H position mors G":dbl, "43 ACH43 b74 Mes Fente V position mors B":dbl, "44 ACH44 b78 Mes position Ecran 2":dbl, "45 ACH45 b80 Mes I obcs Faraday 1":dbl, "46 ACH46 b82 Mes I obcs Faraday 3":dbl, "47 ACH47 b84 Mes position Miroir X":dbl, "48 ACH48 b85 Mes position Miroir Y":dbl, "49 ACH49 b87 Signal laser 2":dbl, "50 ACH50 b89 Libre ?":dbl, "51 ACH51 b91 Libre ?":dbl, "52 ACH52 b93 Libre ?":dbl, "53 ACH53 b95 Libre ?":dbl, "54 ACH54 b97 Libre ?":dbl, "55 ACH55 b99 Libre ?":dbl, "56 ACH56 b86 Signal laser 1":dbl, "57 ACH57 b88 Libre ?":dbl, "58 ACH58 b90 Libre ?":dbl, "59 ACH59 b92 Libre ?":dbl, "60 ACH60 b94 Libre ?":dbl, "61 ACH61 b96 Libre ?":dbl, "62 ACH62 b98 Libre ?":dbl, "63 ACH63 b100 Libre ?":dbl}
  T16 = cluster{"00 APA0 b47 Reffroidissement Canon marche":bool, "01 APA1 b45 Reffroidissement Canon défaut":bool, "02 APA2 b43 Vanne Reffroidissement Canon fermée":bool, "03 APA3 b41 Vanne Reffroidissement Canon ouverte":bool, "04 APA4 b39 Débit Reffroidissement Canon défaut":bool, "05 APA5 b37 Local / Distance Canon (local=0V)":bool, "06 APA6 b35 Reffroidissement Section marche":bool, "07 APA7 b33 Reffroidissement Section défaut":bool, "08 APB0 b31 Vanne Reffroidissement Section fermée":bool, "09 APB1 b29 Vanne Reffroidissement Section ouverte":bool, "10 APB2 b27 Débit eau Reffroidissement Section":bool, "11 APB3 b25 Loc/dist. Reffr. Section (local=0V)":bool, "12 APB4 b23 Triplet 1-1 en marche":bool, "13 APB5 b21 Triplet 1-1 en défaut":bool, "14 APB6 b19 Triplet 1-2 en marche":bool, "15 APB7 b17 Triplet 1-2 en défaut":bool, "16 APC0 b15 Réserve":bool, "17 APC1 b13 Réserve":bool, "18 APC2 b11 Triplet 2-1 en marche":bool, "19 APC3 b09 Triplet 2-1 en défaut":bool, "20 APC4 b07 Triplet 2-2 en marche":bool, "21 APC5 b05 Triplet 2-2 en défaut":bool, "22 APC6 b03 Réserve":bool, "23 APC7 b01 Réserve":bool, "24 BPA0 b48 Quadripôple 1 en marche":bool, "25 BPA1 b46 Quadripôple 1 en défaut":bool, "26 BPA2 b44 Quadripôple 2 en marche":bool, "27 BPA3 b42 Quadripôple 2 en défaut":bool, "28 BPA4 b40 Focale injection en marche":bool, "29 BPA5 b38 Focale injection en défaut":bool, "30 BPA6 b36 eau focale injection en défaut":bool, "31 BPA7 b34 Dipôle 1 en marche":bool, "32 BPB0 b32 Dipôle 1 en défaut":bool, "33 BPB1 b30 Dipôle 2 en marche":bool, "34 BPB2 b28 Dipôle 2 en défaut":bool, "35 BPB3 b26 Guidage H 1 en marche":bool, "36 BPB4 b24 Guidage H 1 en défaut":bool, "37 BPB5 b22 Guidage V 1 en marche":bool, "38 BPB6 b20 Guidage V 1 en défaut":bool, "39 BPB7 b18 Guidage H 2 en marche":bool, "40 BPC0 b16 Guidage H 2 en défaut":bool, "41 BPC1 b14 Guidage V 2 en marche":bool, "42 BPC2 b12 Guidage V 2 en défaut":bool, "43 BPC3 b10 Guidage H 3 en marche":bool, "44 BPC4 b08 Guidage H 3 en défaut":bool, "45 BPC5 b06 Guidage V 3 en marche":bool, "46 BPC6 b04 Guidage V 3 en défaut":bool, "47 BPC7 b02 Guidage H 4 en marche":bool, "48 CPA0 b97 Guidage H 4 en défaut":bool, "49 CPA1 b95 Guidage V 4 en marche":bool, "50 CPA2 b93 Guidage V 4 en défaut":bool, "51 CPA3 b91 Réserve":bool, "52 CPA4 b89 Réserve":bool, "53 CPA5 b87 Guidage V 5 en marche":bool, "54 CPA6 b85 Guidage V 5 en défaut":bool, "55 CPA7 b83 Réserve":bool}
  T17 = cluster{"00 CPB0 b81 Marche Reffroidissement Canon":bool, "01 CPB1 b79 Arrêt Reffroidissement Canon":bool, "02 CPB2 b77 RAZ Reffroidissement Canon":bool, "03 CPB3 b75 Marche Reffroidissement Section":bool, "04 CPB4 b73 Arrêt Reffroidissement Section":bool, "05 CPB5 b71 RAZ Reffroidissement Section":bool, "06 CPB6 b69 Réserve":bool, "07 CPB7 b67 Réserve":bool, "08 CPC0 b65 Réserve":bool, "09 CPC1 b63 Marche Triplet 1-1":bool, "10 CPC2 b61 Réserve":bool, "11 CPC3 b59 Marche Triplet 1-2":bool, "12 CPC4 b57 Réserve":bool, "13 CPC5 b55 Réserve":bool, "14 CPC6 b53 Réserve":bool, "15 CPC7 b51 Marche Triplet 2-1":bool, "16 DPA0 b98 Réserve":bool, "17 DPA1 b96 Marche Triplet 2-2":bool, "18 DPA2 b94 Réserve":bool, "19 DPA3 b92 Réserve":bool, "20 DPA4 b90 Réserve":bool, "21 DPA5 b88 M/A Quadripôple 1":bool, "22 DPA6 b86 Réserve":bool, "23 DPA7 b84 M/A Quadripôple 2":bool, "24 DPB0 b82 Réserve":bool, "25 DPB1 b80 M/A Focale Injection":bool, "26 DPB2 b78 Réserve":bool, "27 DPB3 b76 M/A Dipôle 1":bool, "28 DPB4 b74 Réserve":bool, "29 DPB5 b72 M/A Dipôle 2":bool, "30 DPB6 b70 Réserve":bool, "31 DPB7 b68 M/A Guidage H1":bool, "32 DPC0 b66 M/A Guidage V1":bool, "33 DPC1 b64 M/A Guidage H2":bool, "34 DPC2 b62 M/A Guidage V2":bool, "35 DPC3 b60 M/A Guidage H3":bool, "36 DPC4 b58 M/A Guidage V3":bool, "37 DPC5 b56 M/A Guidage H4":bool, "38 DPC6 b54 M/A Guidage V4":bool, "39 DPC7 b52 M/A Guidage V5":bool}
  T18 = cluster{"00 APA0 b47 Eau corps Klystron":bool, "01 APA1 b45 Eau collecteur Klystron":bool, "02 APA2 b43 Eau cuve Klystron":bool, "03 APA3 b41 Vide Klystron":bool, "04 APA4 b39 Ventilation Thyratron":bool, "05 APA5 b37 Niveau d'huile cuve Klystron":bool, "06 APA6 b35 V chauffage Thyratron":bool, "07 APA7 b33 I chauffage Thyratron":bool, "08 APB0 b31 V chauffage Klystron":bool, "09 APB1 b29 I chauffage Klystron":bool, "10 APB2 b27 I De QING":bool, "11 APB3 b25 I réservoir Thyratron":bool, "12 APB4 b23 Sécurité Thyratron":bool, "13 APB5 b21 Pression SF6":bool, "14 APB6 b19 I prémagnétisation":bool, "15 APB7 b17 Contact porte":bool, "16 APC0 b15 Contact perche":bool, "17 APC1 b13 Contact capot cuve":bool, "18 APC2 b11 Fin Tempo":bool, "19 APC3 b09 Débit eau Canon":bool, "20 APC4 b07 Eau focale Klystron":bool, "21 APC5 b05 I Focale 1":bool, "22 APC6 b03 I Focale 2":bool, "23 APC7 b01 I Focale 3":bool, "24 BPA0 b48 Réserve":bool, "25 BPA1 b46 Réserve":bool, "26 BPA2 b44 Réserve":bool, "27 BPA3 b42 Déphaseur butée MIN":bool, "28 BPA4 b40 Déphaseur butée MAX":bool, "29 BPA5 b38 Atténuateur butée MIN":bool, "30 BPA6 b36 Atténuateur butée MAX":bool, "31 BPA7 b34 Réserve":bool, "32 BPB0 b32 Relais 2 ouvert":bool, "33 BPB1 b30 HF incident Canon":bool, "34 BPB2 b28 HF incident Section":bool, "35 BPB3 b26 V alimentation HT":bool, "36 BPB4 b24 I alimentation HT":bool, "37 BPB5 b22 Relais 1 ouvert":bool, "38 BPB6 b20 Débit eau Section":bool, "39 BPB7 b18 Résistivité":bool, "40 BPC0 b16 Vide Injection":bool, "41 BPC1 b14 I Thyratron":bool, "42 BPC2 b12 I fin de ligne":bool, "43 BPC3 b10 V LAR":bool, "44 BPC4 b08 V Klystron":bool, "45 BPC5 b06 I Klystron":bool, "46 BPC6 b04 Radioprotection 1, coupure HT":bool, "47 BPC7 b02 Radioprotection 2, coupure HF":bool, "48 CPA0 b97 Alimentation HT en marche":bool, "49 CPA1 b95 Alimentation HT en défaut":bool, "50 CPA2 b93 Réserve":bool, "51 CPA3 b91 Réserve":bool, "52 CPA4 b89 Contact porte légère fermée":bool, "53 CPA5 b87 Contact porte lourde fermée":bool, "54 CPA6 b85 Contact porte secours fermée":bool, "55 CPA7 b83 Contact porte laser fermée":bool, "56 CPB0 b81 Totalisation des AU":bool, "57 CPB1 b79 Rondier 1":bool, "58 CPB2 b77 Rondier 2":bool, "59 CPB3 b75 Rondier 3":bool, "60 CPB4 b73 Totalisation des rondiers":bool, "61 CPB5 b71 Position BACO PA / MOD":bool, "62 CPB6 b69 Position BACO de TIR":bool, "63 CPB7 b67 Position occulteur LASER":bool}
  T19 = cluster{"00 CPC0 b65 Marche modulateur Bas Niveau":bool, "01 CPC1 b63 Arrêt modulateur Bas Niveau":bool, "02 CPC2 b61 RAZ modulateur Bas Niveau":bool, "03 CPC3 b59 Marche Chauffage":bool, "04 CPC4 b57 Arrêt Chauffage":bool, "05 CPC5 b55 Marche prémagnétisation":bool, "06 CPC6 b53 Arrêt prémagnétisation":bool, "07 CPC7 b51 Marche focale Klystron":bool, "08 DPA0 b98 Arrêt focale Klystron":bool, "09 DPA1 b96 Réserve":bool, "10 DPA2 b94 Réserve":bool, "11 DPA3 b92 Réserve":bool, "12 DPA4 b90 Réserve":bool, "13 DPA5 b88 Réserve":bool, "14 DPA6 b86 Réserve":bool, "15 DPA7 b84 Réserve":bool, "16 DPB0 b82 Marche relais HT 1":bool, "17 DPB1 b80 Arrêt relais HT 1":bool, "18 DPB2 b78 Marche alimentation HT":bool, "19 DPB3 b76 Arrêt alimentation HT":bool, "20 DPB4 b74 RAZ alimentation HT":bool, "21 DPB5 b72 Réserve":bool, "22 DPB6 b70 Réserve":bool, "23 DPB7 b68 Réserve":bool, "24 DPC0 b66 Réserve":bool, "25 DPC1 b64 Réserve":bool, "26 DPC2 b62 Réserve":bool, "27 DPC3 b60 Réserve":bool, "28 DPC4 b58 Réserve":bool, "29 DPC5 b56 M/A alimentation Att. et Deph.":bool, "30 DPC6 b54 Réserve":bool, "31 DPC7 b52 Réserve":bool}
  T20 = cluster{"00 APA0 b47 Vide chambre préparatoire en marche":bool, "01 APA1 b45 Réserve":bool, "02 APA2 b43 Vide sas guide HF en marche":bool, "03 APA3 b41 Vide sas guide HF en défaut":bool, "04 APA4 b39 Vide Canon (PIQ 12) en marche":bool, "05 APA5 b37 Vide Canon (PIQ 12) en défaut":bool, "06 APA6 b35 Vide Section (PIQ 16) en marche":bool, "07 APA7 b33 Vide Section (PIQ 16) en défaut":bool, "08 APB0 b31 Vide Miroir (PIQ 21) en marche":bool, "09 APB1 b29 Vide Miroir (PIQ 21) en défaut":bool, "10 APB2 b27 Vide Dipôle 1 (PIQ 27+33) en marche":bool, "11 APB3 b25 Vide Dipôle 1 (PIQ 27+33) en défaut":bool, "12 APB4 b23 Vide Ecran 1 (PIQ 53+63) en marche":bool, "13 APB5 b21 Vide Ecran 1 (PIQ 53+63) en défaut":bool, "14 APB6 b19 Vanne Cathode (VIC 01) ouverte":bool, "15 APB7 b17 Vanne Cathode (VIC 01) fermée":bool, "16 APC0 b15 Vanne Injection (VSC 17) ouverte":bool, "17 APC1 b13 Vanne Injection (VSC 17) fermée":bool, "18 APC2 b11 Vanne directe ouverte":bool, "19 APC3 b09 Vanne directe fermée":bool, "20 APC4 b07 Vanne Déviation 1 ouverte":bool, "21 APC5 b05 Vanne Déviation 1 fermée":bool, "22 APC6 b03 Vanne Déviation 2 ouverte":bool, "23 APC7 b01 Vanne Déviation 2 fermée":bool, "24 BPA0 b48 LASER en marche":bool, "25 BPA1 b46 LASER eb défaut":bool, "26 BPA2 b44 Réserve":bool, "27 BPA3 b42 Réserve":bool, "28 BPA4 b40 Réserve":bool, "29 BPA5 b38 Réserve":bool, "30 BPA6 b36 Réserve":bool, "31 BPA7 b34 Réserve":bool, "32 BPB0 b32 Réserve":bool, "33 BPB1 b30 Réserve":bool, "34 BPB2 b28 Réserve":bool, "35 BPB3 b26 Réserve":bool, "36 BPB4 b24 Réserve":bool, "37 BPB5 b22 Faraday 1 EN":bool, "38 BPB6 b20 Faraday 1 HORS":bool, "39 BPB7 b18 Faraday 2 EN":bool, "40 BPC0 b16 Faraday 2 HORS":bool, "41 BPC1 b14 Faraday 3 HORS":bool, "42 BPC2 b12 Faraday 3 EN":bool, "43 BPC3 b10 Position Miroir LASER EN":bool, "44 BPC4 b08 Position Miroir LASER HORS":bool, "45 BPC5 b06 Fente H butée MIN":bool, "46 BPC6 b04 Mors HG butée HORS":bool, "47 BPC7 b02 Mors HD butée HORS":bool, "48 CPA0 b97 Réserve":bool, "49 CPA1 b95 Réserve":bool, "50 CPA2 b93 Translateur écran 1 en défaut":bool, "51 CPA3 b91 Translateur écran 2 en défaut":bool, "52 CPA4 b89 Translateur écran 3 en défaut":bool, "53 CPA5 b87 Réserve":bool, "54 CPA6 b85 Réserve":bool, "55 CPA7 b83 Réserve":bool}
  T21 = cluster{"00 CPB0 b81 Réserve":bool, "01 CPB1 b79 Alimentation moteur":bool, "02 CPB2 b77 Réserve":bool, "03 CPB3 b75 M/A Caméra chambre de préparation":bool, "04 CPB4 b73 Réserve":bool, "05 CPB5 b71 M/A Caméra Miroir":bool, "06 CPB6 b69 Réserve":bool, "07 CPB7 b67 M/A Eclairage Ecran 1":bool, "08 CPC0 b65 Réserve":bool, "09 CPC1 b63 M/A Caméra Ecran 1":bool, "10 CPC2 b61 Réserve":bool, "11 CPC3 b59 Réserve":bool, "12 CPC4 b57 Réserve":bool, "13 CPC5 b55 M/A Eclairage Ecran 2":bool, "14 CPC6 b53 Réserve":bool, "15 CPC7 b51 M/A Caméra Ecran 2":bool, "16 DPA0 b98 Réserve":bool, "17 DPA1 b96 Réserve":bool, "18 DPA2 b94 Réserve":bool, "19 DPA3 b92 M/A Eclairage Ecran 3":bool, "20 DPA4 b90 Réserve":bool, "21 DPA5 b88 M/A Caméra Ecran 3":bool, "22 DPA6 b86 Cmd Miroir LASER EN":bool, "23 DPA7 b84 Cmd Faraday 1 EN":bool, "24 DPB0 b82 Cmd Faraday 2 EN":bool, "25 DPB1 b80 Cmd Faraday 3 EN":bool, "26 DPB2 b78 Cmd Miroir LASER HORS":bool, "27 DPB3 b76 M/A alimentation Fente H":bool, "28 DPB4 b74 Cmd Faraday 1 HORS":bool, "29 DPB5 b72 Cmd Faraday 2 HORS":bool, "30 DPB6 b70 Cmd Faraday 3 HORS":bool, "31 DPB7 b68 M/A Alimentation Ecrans":bool, "32 DPC0 b66 LASER Marche":bool, "33 DPC1 b64 LASER Arrêt":bool, "34 DPC2 b62 Réserve":bool, "35 DPC3 b60 Réserve":bool, "36 DPC4 b58 Réserve":bool, "37 DPC5 b56 Réserve":bool, "38 DPC6 b54 Réserve":bool, "39 DPC7 b52 Réserve":bool}
  T22 = cluster{"00 OUT00 b01 Cmd Guidage H1":dbl, "01 OUT01 b05 Cmd Guidage V1":dbl, "02 OUT02 b09 Cmd Guidage H2":dbl, "03 OUT03 b13 Cmd Guidage V2":dbl, "04 OUT04 b17 Cmd Guidage H3":dbl, "05 OUT05 b21 Cmd Guidage V3":dbl, "06 OUT06 b25 Cmd Guidage H4":dbl, "07 OUT07 b29 Cmd Guidage V4":dbl, "08 OUT08 b33 Réserve":dbl, "09 OUT09 b37 Cmd Guidage V5":dbl}
  T23 = cluster{"00 OUT00 b01 Cmd I Triplet 1-1":dbl, "01 OUT01 b05 Cmd I Triplet 1-2":dbl, "02 OUT02 b09 Réserve":dbl, "03 OUT03 b13 Cmd I Triplet 2-1":dbl, "04 OUT04 b17 Cmd I Triplet 2-2":dbl, "05 OUT05 b21 Cmd I Solénoïde":dbl, "06 OUT06 b25 Cmd I Quad 1":dbl, "07 OUT07 b29 Cmd I Quad 2":dbl, "08 OUT08 b33 Cmd I Dipôle 1":dbl, "09 OUT09 b37 Cmd I Dipôle 2":dbl}
  T24 = cluster{"00 OUT00 b01 Réserve":dbl, "01 OUT01 b05 Cmd Temp. Canon":dbl, "02 OUT02 b09 Cmd Temp. Section":dbl, "03 OUT03 b13 Cmd Pos. Déphaseur":dbl, "04 OUT04 b17 Cmd Pos. Atténuateur":dbl, "05 OUT05 b21 Cmd déphasage HF/LASER":dbl, "06 OUT06 b25 Cmd amplitude HF préampli":dbl, "07 OUT07 b29 Réserve":dbl, "08 OUT08 b33 Cmd position Miroir X":dbl, "09 OUT09 b37 Cmd position Miroir Y":dbl}
  T25 = cluster{"00 OUT00 b01 Cmd alimentation HT":dbl, "01 OUT01 b05 Cmd DeQing":dbl, "02 OUT02 b09 Cmd position fente HG":dbl, "03 OUT03 b13 Cmd position fente HD":dbl, "04 OUT04 b17 Cmd position translateur Ecran 1":dbl, "05 OUT05 b21 Cmd position translateur Ecran 2":dbl, "06 OUT06 b25 Cmd position translateur Ecran 3":dbl, "07 OUT07 b29 Réserve":dbl, "08 OUT08 b33 Réserve":dbl, "09 OUT09 b37 Réserve":dbl}
  T26 = cluster{"00 OUT00 b05 C10 Délais":dbl, "01 OUT00 b05 C10 Largeur":dbl, "02 OUT01 b09 C10 Délais":dbl, "03 OUT01 b09 C10 Largeur":dbl, "04 OUT02 b32 C10 Délais":dbl, "05 OUT02 b32 C10 Largeur":dbl, "06 OUT03 b29 C10 Délais":dbl, "07 OUT03 b29 C10 Largeur":dbl, "08 OUT04 b26 C10 Délais":dbl, "09 OUT04 b26 C10 Largeur":dbl, "10 OUT05 b23 C10 Délais":dbl, "11 OUT05 b23 C10 Largeur":dbl, "12 OUT06 b53 C10 Délais":dbl, "13 OUT06 b53 C10 Largeur":dbl, "14 OUT07 b16 C10 Délais":dbl, "15 OUT07 b16 C10 Largeur":dbl, "16 OUT00 b05 C11 Délais":dbl, "17 OUT00 b05 C11 Largeur":dbl, "18 OUT01 b09 C11 Délais":dbl, "19 OUT01 b09 C11 Largeur":dbl, "20 OUT02 b32 C11 Délais":dbl, "21 OUT02 b32 C11 Largeur":dbl, "22 OUT03 b29 C11 Délais":dbl, "23 OUT03 b29 C11 Largeur":dbl, "24 OUT04 b26 C11 Délais":dbl, "25 OUT04 b26 C11 Largeur":dbl, "26 OUT05 b23 C11 Délais":dbl, "27 OUT05 b23 C11 Largeur":dbl, "28 OUT06 b53 C11 Délais":dbl, "29 OUT06 b53 C11 Largeur":dbl, "30 OUT07 b16 C11 Délais":dbl, "31 OUT07 b16 C11 Largeur":dbl, "N° du compteur":dbl}
  T27 = cluster{"-":bool, "-":bool, "-":bool, "-":bool, "-":bool, "-":bool, "-":bool, "-":bool, "-":bool, "-":bool, "-":bool, "-":bool, "-":bool, "-":bool, "-":bool, "-":bool, "-":bool, "-":bool, "-":bool, "-":bool, "-":bool, "-":bool, "-":bool, "-":bool, "-":bool, "-":bool, "-":bool, "-":bool, "-":bool, "-":bool, "-":bool, "-":bool, "-":bool, "-":bool, "-":bool, "-":bool, "-":bool, "-":bool, "-":bool, "-":bool, "-":bool, "-":bool, "-":bool, "-":bool, "-":bool, "-":bool, "-":bool, "-":bool, "-":bool, "-":bool, "-":bool, "-":bool, "-":bool, "-":bool, "-":bool, "-":bool, "-":bool, "-":bool, "-":bool, "-":bool, "-":bool, "-":bool, "-":bool, "-":bool, "-":bool, "-":bool, "-":bool, "-":bool, "-":bool, "-":bool, "-":bool, "-":bool, "-":bool, "-":bool, "-":bool, "-":bool, "-":bool, "-":bool, "-":bool, "-":bool}
  T28 = cluster{"Pilote présent ?":bool, "-":bool, "-":bool, "-":bool, "-":bool, "-":bool, "-":bool, "-":bool, "-":bool, "-":bool, "-":bool, "-":bool, "-":bool, "-":bool, "-":bool, "-":bool, "-":bool, "-":bool, "-":bool, "-":bool, "-":bool, "-":bool, "-":bool, "-":bool, "-":bool, "-":bool, "-":bool, "-":bool, "-":bool, "-":bool, "-":bool, "-":bool, "-":bool, "-":bool, "-":bool, "-":bool, "-":bool, "-":bool, "-":bool, "-":bool, "-":bool, "-":bool, "-":bool, "-":bool, "-":bool, "-":bool, "-":bool, "-":bool, "-":bool, "-":bool, "-":bool, "-":bool, "-":bool, "-":bool, "-":bool, "-":bool, "-":bool, "-":bool, "-":bool, "-":bool, "-":bool, "-":bool, "-":bool, "-":bool, "-":bool, "-":bool, "-":bool, "-":bool, "-":bool, "-":bool, "-":bool, "-":bool, "-":bool, "-":bool, "-":bool, "-":bool, "-":bool, "-":bool, "-":bool, "-":bool}
  T29 = cluster{"00 SUP Vidéo":dbl, "01 SUP Variables":dbl, "02 SUP Evenement":dbl, "03":dbl, "04":dbl, "05":dbl, "06":dbl, "07":dbl, "08":dbl, "09":dbl, "10":dbl, "11":dbl, "12":dbl, "13":dbl, "14":dbl, "15":dbl, "16":dbl, "17":dbl, "18":dbl, "19":dbl, "20":dbl, "21":dbl, "22":dbl, "23":dbl, "24":dbl, "25":dbl, "26":dbl, "27":dbl, "28":dbl, "29":dbl, "30":dbl, "31":dbl, "32":dbl, "33":dbl, "34":dbl, "35":dbl, "36":dbl, "37":dbl, "38":dbl, "39":dbl, "40":dbl, "41":dbl, "42":dbl, "43":dbl, "44":dbl, "45":dbl, "46":dbl, "47":dbl, "48":dbl, "49":dbl, "50":dbl, "51":dbl, "52":dbl, "53":dbl, "54":dbl, "55":dbl, "56":dbl, "57":dbl, "58":dbl, "59":dbl, "60":dbl, "61":dbl, "62":dbl, "63":dbl}
  T30 = cluster{"00 ACQ Auxiliare":dbl, "01 ACQ Variables":dbl, "02 ACQ Evénement":dbl, "03 ":dbl, "04":dbl, "05":dbl, "06":dbl, "07":dbl, "08":dbl, "09":dbl, "10 ACQ Vide Section":dbl, "11 ACQ Vide Chambre":dbl, "12 ACQ Vide PI Guide HF":dbl, "13 ACQ Vide Canon PIQ12":dbl, "14 ACQ Vide Section PIQ16":dbl, "15 ACQ Vide Miroir PIQ21":dbl, "16 ACQ Vide Dip PIQ27/33 ":dbl, "17 ACQ Vide Ecran PIQ53/63":dbl, "18 ACQ Libre":dbl, "19 ACQ Libre":dbl, "20 ACQ Vide TPG300 PIQ63":dbl, "21":dbl, "22":dbl, "23":dbl, "24":dbl, "25":dbl, "26":dbl, "27":dbl, "28":dbl, "29":dbl, "30":dbl, "31":dbl, "32 WCM2HMax":dbl, "33 WCM2BMax":dbl, "34 WCM2GMax":dbl, "35 WCM2DMax":dbl, "36 WCM2HMin":dbl, "37 WCM2BMin":dbl, "38 WCM2GMin":dbl, "39 WCM2DMin":dbl, "40":dbl, "41":dbl, "42":dbl, "43":dbl, "44":dbl, "45":dbl, "46":dbl, "47":dbl, "48":dbl, "49":dbl, "50":dbl, "51":dbl, "52":dbl, "53":dbl, "54":dbl, "55":dbl, "56":dbl, "57":dbl, "58":dbl, "59":dbl, "60":dbl, "61":dbl, "62":dbl, "63 B_NI6220":dbl}
  T31 = cluster{"00":dbl, "01":dbl, "02":dbl, "03":dbl, "04":dbl, "05":dbl, "06":dbl, "07":dbl, "08":dbl, "09":dbl, "10":dbl, "11":dbl, "12":dbl, "13":dbl, "14":dbl, "15":dbl, "16":dbl, "17":dbl, "18":dbl, "19":dbl, "20":dbl, "21":dbl, "22":dbl, "23":dbl, "24":dbl, "25":dbl, "26":dbl, "27":dbl, "28":dbl, "29":dbl, "30":dbl, "31":dbl, "32":dbl, "33":dbl, "34":dbl, "35":dbl, "36":dbl, "37":dbl, "38":dbl, "39":dbl, "40":dbl, "41":dbl, "42":dbl, "43":dbl, "44":dbl, "45":dbl, "46":dbl, "47":dbl, "48":dbl, "49":dbl, "50":dbl, "51":dbl, "52":dbl, "53":dbl, "54":dbl, "55":dbl, "56":dbl, "57":dbl, "58":dbl, "59":dbl, "60":dbl, "61":dbl, "62":dbl, "63":dbl}
  T32 = cluster{"Read Access":enum8{"Allowed", "Required", "Denied"}, "Write Access":enum8{"Allowed", "Required", "Denied"}}
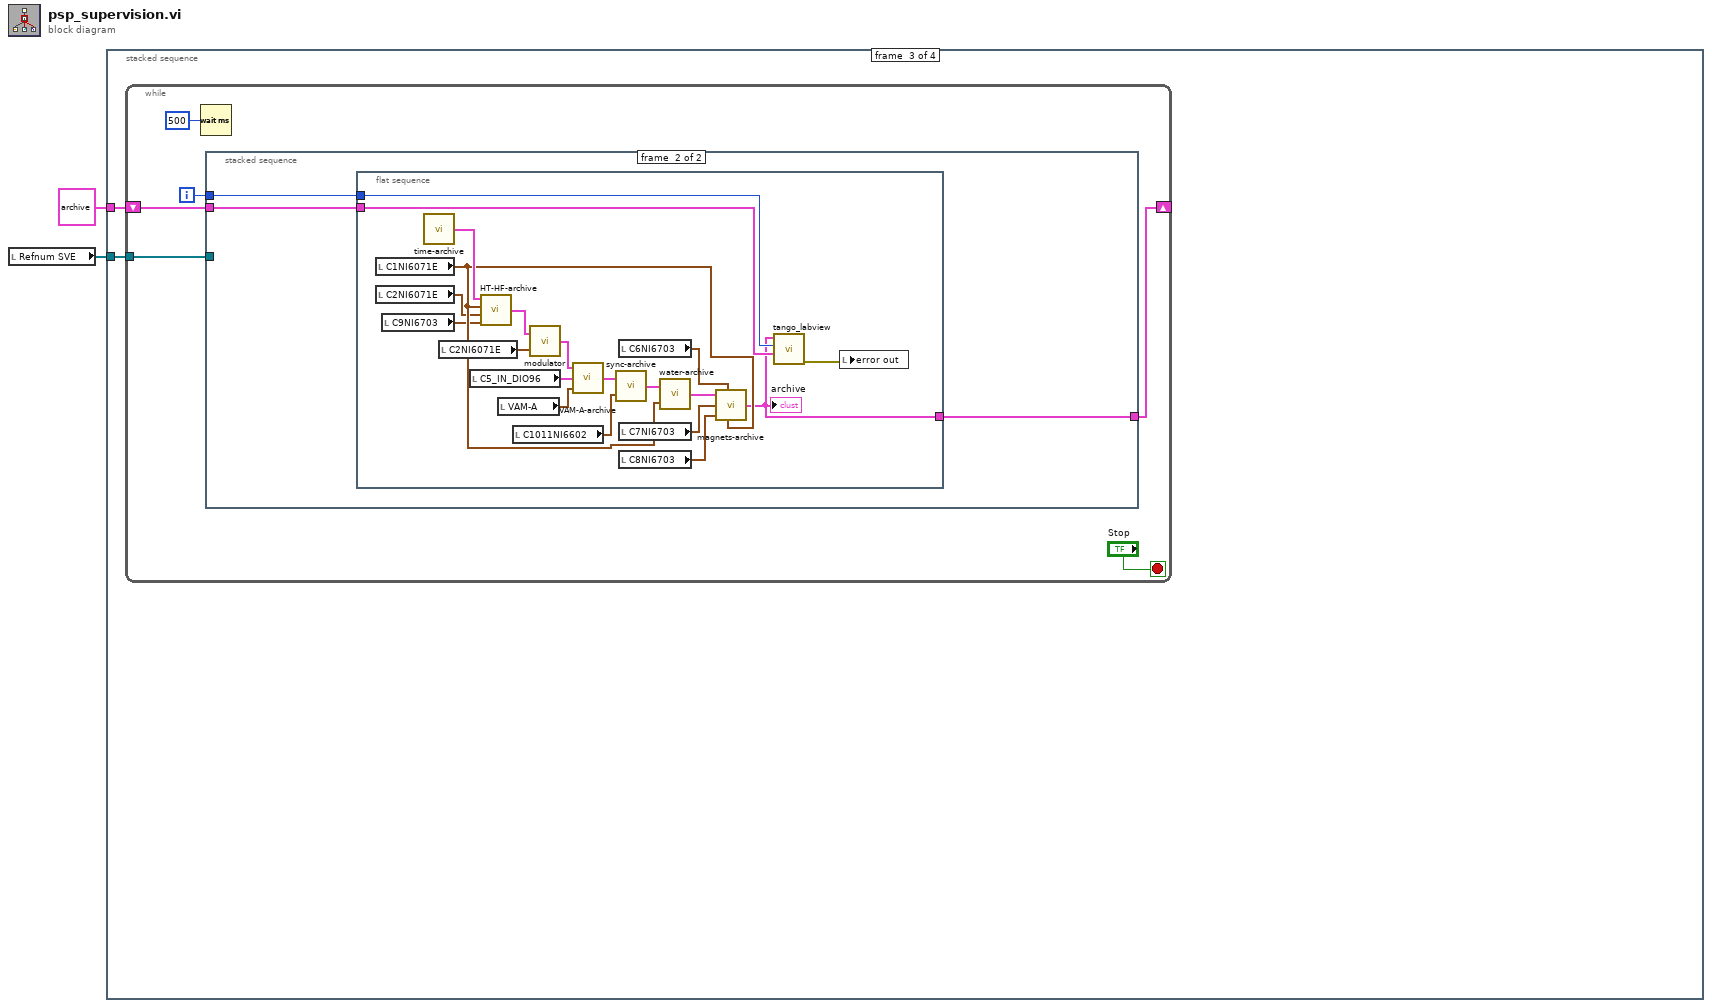
[diagram p0: block diagram]
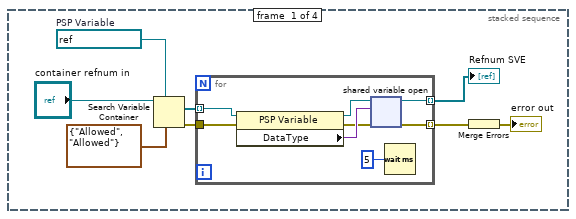
[diagram p2: hidden frame]
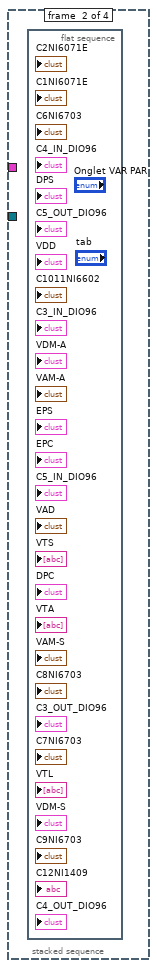
[diagram p3: hidden frame]
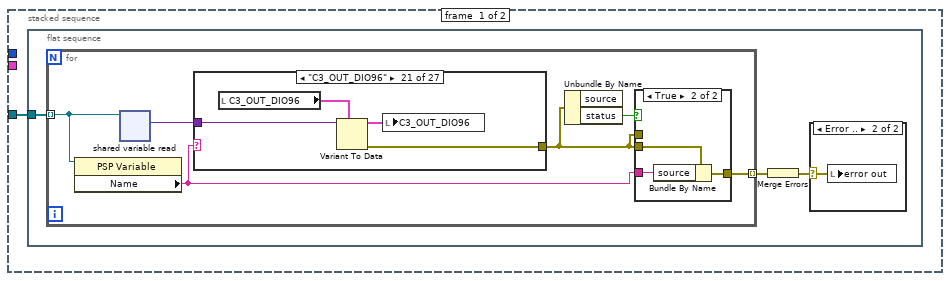
[diagram p4: hidden frame]
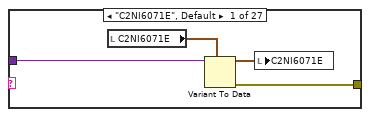
[diagram p7: hidden frame]
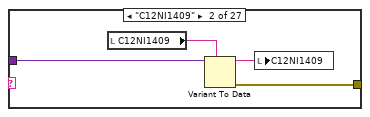
[diagram p8: hidden frame]
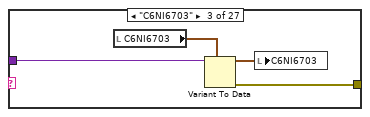
[diagram p9: hidden frame]
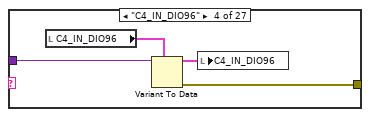
[diagram p10: hidden frame]
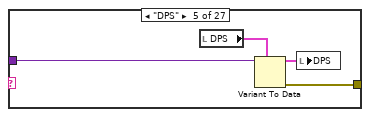
[diagram p11: hidden frame]
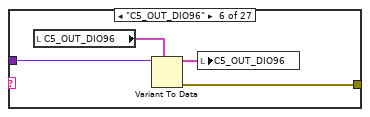
[diagram p12: hidden frame]
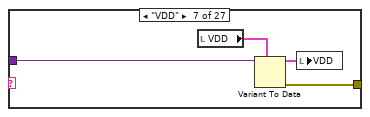
[diagram p13: hidden frame]
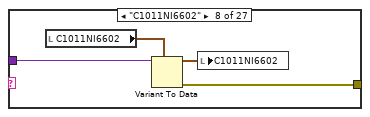
[diagram p14: hidden frame]
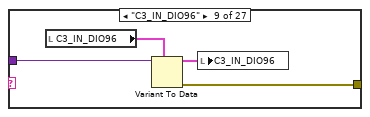
[diagram p15: hidden frame]
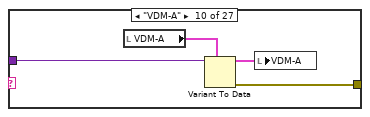
[diagram p16: hidden frame]
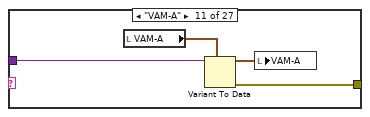
[diagram p17: hidden frame]
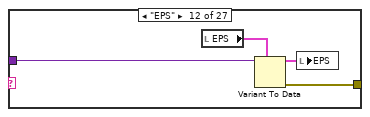
[diagram p18: hidden frame]
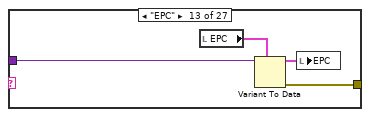
[diagram p19: hidden frame]
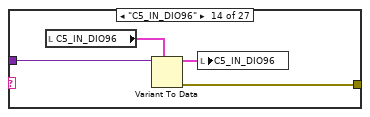
[diagram p20: hidden frame]
diagram:
  n1 = local read "Refnum SVE"() -> (w2:refnum<k21>[])
  n2 = stacked-sequence {
    tunnel: w2 -> [_ _ w20 w173]
    tunnel: T1 {"sync"={"elyse/sync/NI6071E/delay"=0.0, "elyse/sync/NI6071E/width"=0.0, "elyse/sync/frequency/delay"=0.0, "elyse/sync/frequency/width"=0.0, "elyse/sync/WCM/delay"=0.0, "elyse/sync/WCM/width"=0.0, "elyse/sync/modulator/delay"=0.0, "elyse/sync/modulator/width"=0.0, "elyse/sync/HF/delay"=0.0, "elyse/sync/HF/width"=0.0, "elyse/sync/Faraday/delay"=0.0, "elyse/sync/Faraday/width"=0.0, "elyse/sync/Oscilloscope/delay"=0.0, "elyse/sync/Oscilloscope/width"=0.0, "elyse/sync/50Hz_20MHz/delay"=0.0, "elyse/sync/50Hz_20MHz/width"=0.0, "elyse/sync/laser_HF/delay"=0.0, "elyse/sync/laser_HF/width"=0.0, "elyse/sync/IMAC/delay"=0.0, "elyse/sync/IMAC/width"=0.0, "elyse/sync/laser/delay"=0.0, "elyse/sync/laser/width"=0.0, "elyse/sync/oscilloscope1/delay"=0.0, "elyse/sync/oscilloscope1/width"=0.0, "elyse/sync/oscilloscope2/delay"=0.0, "elyse/sync/oscilloscope2/width"=0.0, "elyse/sync/detection1/delay"=0.0, "elyse/sync/detection1/width"=0.0, "elyse/sync/detection1/delay"=0.3, "elyse/sync/detection2/width"=0.0, "elyse/sync/machine/delay"=0.0, "elyse/sync/machine/width"=0.0, "elyse/sync/n_selection"=0.0}, "HT"={"elyse/HT/voltage/set_value"=0.0, "elyse/HT/voltage/value"=0.0, "elyse/HT/current/value"=0.0, "elyse/preamplifier/set_value"=0.0, "elyse/preamplifier/value"=0.0}, "HF"={"elyse/HF/attenuator/value"=25.43007170139925, "elyse/HF/dephaser/value"=102.28, "elyse/HF/dephaser/value_manuel"=102.28, "elyse/HF/canon/value"=0.0, "elyse/HF/section/value"=0.0}, "vacuum"={"elyse/vacuum/preparation_chamber/state"=FALSE, "elyse/vacuum/preparation_chamber/measurement"=0.0, "elyse/vacuum/HF/state"=FALSE, "elyse/vacuum/HF/measurement"=1.0399999999999999e-08, "elyse/vacuum/canon/state"=FALSE, "elyse/vacuum/canon/measurement"=6.1e-09, "elyse/vacuum/section/state"=FALSE, "elyse/vacuum/section/measurement"=6e-09, "elyse/vacuum/dipole1/state"=FALSE, "elyse/vacuum/dipole1/measurement"=2.7e-09, "elyse/vacuum/screen1/state"=FALSE, "elyse/vacuum/screen1/measurement"=2.2e-09, "elyse/vacuum/mirror/state"=FALSE, "elyse/vacuum/mirror/measurement"=3.5999999999999996e-09, "elyse/vacuum/tpg300_section/state"=FALSE, "elyse/vacuum/tpg300_section/measurement"=0.0, "elyse/vacuum/valves/cathode/state"=FALSE, "elyse/vacuum/valves/injection/state"=FALSE}, "modulator"={"elyse/modulator/focale1/current/value"=0.0, "elyse/modulator/focale2/current/value"=0.0, "elyse/modulator/focale3/current/value"=0.0, "elyse/modulator/LAR/voltage/value"=0.0, "elyse/modulator/line_end/current/value"=0.0, "elyse/modulator/thyratron/currents/power/value"=0.0, "elyse/modulator/thyratron_reservoir/current/value"=0.0, "elyse/modulator/paramagnetization/current/value"=0.0, "elyse/modulator/thyratron/voltages/heating/value"=0.0, "elyse/modulator/thyratron/currents/heating/value"=0.0, "elyse/modulator/klystron/currents/power/value"=0.0, "elyse/modulator/klystron/voltages/power/value"=0.0, "elyse/modulator/klystron/currents/heating/value"=0.0, "elyse/modulator/klystron/voltages/heating/value"=0.0}, "cooling"={"elyse/cooling/section/temperature/set_value"=28.0, "elyse/cooling/section/temperature/measurement"=0.0, "elyse/cooling/canon/temperature/set_value"=20.2, "elyse/cooling/canon/temperature/measurement"=0.0}, "magnets"={"elyse/magnets/focale/set_value"=0.0, "elyse/magnets/focale/value"=0.0, "elyse/magnets/phase_HF_laser/set_value"=0.0, "elyse/magnets/phase_HF_laser/value"=0.0, "elyse/magnets/dipole1/set_value"=0.0, "elyse/magnets/dipole1/value"=0.0, "elyse/magnets/dipole2/set_value"=0.0, "elyse/magnets/dipole2/value"=0.0, "elyse/magnets/Cor_H1/set_value"=0.0, "elyse/magnets/Cor_H1/value"=0.0, "elyse/magnets/Cor_V1/set_value"=0.0, "elyse/magnets/Cor_V1/value"=0.0, "elyse/magnets/Cor_H2/set_value"=0.0, "elyse/magnets/Cor_H2/value"=0.0, "elyse/magnets/Cor_V2/set_value"=0.0, "elyse/magnets/Cor_V2/value"=0.0, "elyse/magnets/Cor_H3/set_value"=0.0, "elyse/magnets/Cor_H3/value"=0.0, "elyse/magnets/Cor_V3/set_value"=-5.0, "elyse/magnets/Cor_V3/value"=0.0, "elyse/magnets/Cor_H4/set_value"=0.0, "elyse/magnets/Cor_H4/value"=0.0, "elyse/magnets/Cor_V4/set_value"=0.0, "elyse/magnets/Cor_V4/value"=0.0, "elyse/magnets/Cor_H5/set_value"=0.0, "elyse/magnets/Cor_H5/value"=0.0, "elyse/magnets/Cor_V5/set_value"=0.0, "elyse/magnets/Cor_V5/value"=0.0, "elyse/magnets/triplet1-1/set_value"=0.0, "elyse/magnets/triplet1-1/value"=0.0, "elyse/magnets/triplet1-2/set_value"=0.0, "elyse/magnets/triplet1-2/value"=0.0, "elyse/magnets/triplet2-1/set_value"=0.0, "elyse/magnets/triplet2-1/value"=0.0, "elyse/magnets/triplet2-2/set_value"=0.0, "elyse/magnets/triplet2-2/value"=0.0, "elyse/magnets/qudrupole1/set_value"=0.0, "elyse/magnets/qudrupole1/value"=0.0, "elyse/magnets/qudrupole2/set_value"=0.0, "elyse/magnets/qudrupole2/value"=0.0}, "time"={"elyse/timestamp"=3734415489.2294674}} ("archive") -> [_ _ w19 _]
    frame #0 {
      w5 = refnum<k21> refnum  # PSP Variable
      n3 = Search Variable Container(6:T32 {"Read Access"=enum."Allowed", "Write Access"=enum."Allowed"} ("access type"), 7:w5, 11:"container refnum in") -> (0:w8:errorcluster, 2:w7:refnum<k21>[])  [unwired: 3 in, 1 out]
      n4 = for {
        tunnel: w7 -> [w18] mode=indexing
        tunnel: w8 -> [w17]
        tunnel: [w13] -> w9 mode=indexing
        tunnel: [w12] -> w10 mode=indexing
        n5 = property class="PSP Variable"(reference=w18, error in=w17) -> (reference out=w15:refnum<k21>, error out=w14:errorcluster, "DataType"=w16:variant)
        n6 = shared-variable-open(w15, w14, w16) -> (w12:refnum<k21>, w13:errorcluster)  [unwired: 1 in]
        n7 = Wait (ms)(milliseconds to wait=u32 5) -> ()  [unwired: 1 out]
      }
      "Refnum SVE" <- w10
      n8 = Merge Errors(w9) -> (→"error out":errorcluster)
    }
    frame #1 {
      n9 = flat-sequence {
        frame #0 {
        }
      }
    }
    frame #2 {
      n10 = while {
        tunnel: w20 -> [w24]
        shift-right: [w21] -> _
        shift-left: w19 -> [w22]
        i -> [w23]
        stop <- "Stop" stop-if-true
        n11 = Wait (ms)(milliseconds to wait=u32 500) -> ()  [unwired: 1 out]
        n12 = stacked-sequence {
          tunnel: w24 -> [w27 _]
          tunnel: w23 -> [_ w152]
          tunnel: w22 -> [_ w151]
          tunnel: [_ w150] -> w21
          frame #0 {
            n13 = flat-sequence {
              tunnel: w27 -> [w30]
              frame #0 {
                n14 = for {
                  tunnel: w30 -> [w37] mode=indexing
                  tunnel: [w32] -> w29 mode=indexing
                  n15 = property class="PSP Variable"(reference=w37) -> ("Name"=w33:string)  [unwired: 1 in, 2 out]
                  n16 = shared-variable-read(w37) -> (w36:variant)  [unwired: 1 in, 3 out]
                  n17 = case shown="\"C3_OUT_DIO96\"" w33 {
                    tunnel: w36 -> [w45 w49 w53 w57 w61 w65 w69 w73 w77 w81 w85 w89 w93 w97 w101 w105 w109 w113 w117 w121 w125 w129 w133 w137 w141 w145 w149]
                    tunnel: [w42 w46 w50 w54 w58 w62 w66 w70 w74 w78 w82 w86 w90 w94 w98 w102 w106 w110 w114 w118 w122 w126 w130 w134 w138 w142 w146] -> w34
                    frame "C2NI6071E", Default {
                      n18 = local read "C2NI6071E"() -> (w44:T15)
                      n19 = Variant To Data(type=w44, Variant=w45) -> (data=w43:T15, error out=w42:errorcluster)  [unwired: 1 in]
                      n20 = local write "C2NI6071E"(w43) -> ()
                    }
                    frame "C12NI1409" {
                      n21 = local read "C12NI1409"() -> (w48:string)
                      n22 = Variant To Data(type=w48, Variant=w49) -> (data=w47:string, error out=w46:errorcluster)  [unwired: 1 in]
                      n23 = local write "C12NI1409"(w47) -> ()
                    }
                    frame "C6NI6703" {
                      n24 = local read "C6NI6703"() -> (w52:T22)
                      n25 = Variant To Data(type=w52, Variant=w53) -> (data=w51:T22, error out=w50:errorcluster)  [unwired: 1 in]
                      n26 = local write "C6NI6703"(w51) -> ()
                    }
                    frame "C4_IN_DIO96" {
                      n27 = local read "C4_IN_DIO96"() -> (w56:T18)
                      n28 = Variant To Data(type=w56, Variant=w57) -> (data=w55:T18, error out=w54:errorcluster)  [unwired: 1 in]
                      n29 = local write "C4_IN_DIO96"(w55) -> ()
                    }
                    frame "DPS" {
                      n30 = local read "DPS"() -> (w60:T10)
                      n31 = Variant To Data(type=w60, Variant=w61) -> (data=w59:T10, error out=w58:errorcluster)  [unwired: 1 in]
                      n32 = local write "DPS"(w59) -> ()
                    }
                    frame "C5_OUT_DIO96" {
                      n33 = local read "C5_OUT_DIO96"() -> (w64:T21)
                      n34 = Variant To Data(type=w64, Variant=w65) -> (data=w63:T21, error out=w62:errorcluster)  [unwired: 1 in]
                      n35 = local write "C5_OUT_DIO96"(w63) -> ()
                    }
                    frame "VDD" {
                      n36 = local read "VDD"() -> (w68:T27)
                      n37 = Variant To Data(type=w68, Variant=w69) -> (data=w67:T27, error out=w66:errorcluster)  [unwired: 1 in]
                      n38 = local write "VDD"(w67) -> ()
                    }
                    frame "C1011NI6602" {
                      n39 = local read "C1011NI6602"() -> (w72:T26)
                      n40 = Variant To Data(type=w72, Variant=w73) -> (data=w71:T26, error out=w70:errorcluster)  [unwired: 1 in]
                      n41 = local write "C1011NI6602"(w71) -> ()
                    }
                    frame "C3_IN_DIO96" {
                      n42 = local read "C3_IN_DIO96"() -> (w76:T16)
                      n43 = Variant To Data(type=w76, Variant=w77) -> (data=w75:T16, error out=w74:errorcluster)  [unwired: 1 in]
                      n44 = local write "C3_IN_DIO96"(w75) -> ()
                    }
                    frame "VDM-A" {
                      n45 = local read "VDM-A"() -> (w80:T28)
                      n46 = Variant To Data(type=w80, Variant=w81) -> (data=w79:T28, error out=w78:errorcluster)  [unwired: 1 in]
                      n47 = local write "VDM-A"(w79) -> ()
                    }
                    frame "VAM-A" {
                      n48 = local read "VAM-A"() -> (w84:T30)
                      n49 = Variant To Data(type=w84, Variant=w85) -> (data=w83:T30, error out=w82:errorcluster)  [unwired: 1 in]
                      n50 = local write "VAM-A"(w83) -> ()
                    }
                    frame "EPS" {
                      n51 = local read "EPS"() -> (w88:T11)
                      n52 = Variant To Data(type=w88, Variant=w89) -> (data=w87:T11, error out=w86:errorcluster)  [unwired: 1 in]
                      n53 = local write "EPS"(w87) -> ()
                    }
                    frame "EPC" {
                      n54 = local read "EPC"() -> (w92:T13)
                      n55 = Variant To Data(type=w92, Variant=w93) -> (data=w91:T13, error out=w90:errorcluster)  [unwired: 1 in]
                      n56 = local write "EPC"(w91) -> ()
                    }
                    frame "C5_IN_DIO96" {
                      n57 = local read "C5_IN_DIO96"() -> (w96:T20)
                      n58 = Variant To Data(type=w96, Variant=w97) -> (data=w95:T20, error out=w94:errorcluster)  [unwired: 1 in]
                      n59 = local write "C5_IN_DIO96"(w95) -> ()
                    }
                    frame "VAD" {
                      n60 = local read "VAD"() -> (w100:T31)
                      n61 = Variant To Data(type=w100, Variant=w101) -> (data=w99:T31, error out=w98:errorcluster)  [unwired: 1 in]
                      n62 = local write "VAD"(w99) -> ()
                    }
                    frame "VTS" {
                      n63 = local read "VTS"() -> (w104:string[])
                      n64 = Variant To Data(type=w104, Variant=w105) -> (data=w103:string[], error out=w102:errorcluster)  [unwired: 1 in]
                      n65 = local write "VTS"(w103) -> ()
                    }
                    frame "DPC" {
                      n66 = local read "DPC"() -> (w108:T12)
                      n67 = Variant To Data(type=w108, Variant=w109) -> (data=w107:T12, error out=w106:errorcluster)  [unwired: 1 in]
                      n68 = local write "DPC"(w107) -> ()
                    }
                    frame "VTA" {
                      n69 = local read "VTA"() -> (w112:string[])
                      n70 = Variant To Data(type=w112, Variant=w113) -> (data=w111:string[], error out=w110:errorcluster)  [unwired: 1 in]
                      n71 = local write "VTA"(w111) -> ()
                    }
                    frame "VAM-S" {
                      n72 = local read "VAM-S"() -> (w116:T29)
                      n73 = Variant To Data(type=w116, Variant=w117) -> (data=w115:T29, error out=w114:errorcluster)  [unwired: 1 in]
                      n74 = local write "VAM-S"(w115) -> ()
                    }
                    frame "C8NI6703" {
                      n75 = local read "C8NI6703"() -> (w120:T24)
                      n76 = Variant To Data(type=w120, Variant=w121) -> (data=w119:T24, error out=w118:errorcluster)  [unwired: 1 in]
                      n77 = local write "C8NI6703"(w119) -> ()
                    }
                    frame "C3_OUT_DIO96" {
                      n78 = local read "C3_OUT_DIO96"() -> (w124:T17)
                      n79 = Variant To Data(type=w124, Variant=w125) -> (data=w123:T17, error out=w122:errorcluster)  [unwired: 1 in]
                      n80 = local write "C3_OUT_DIO96"(w123) -> ()
                    }
                    frame "C7NI6703" {
                      n81 = local read "C7NI6703"() -> (w128:T23)
                      n82 = Variant To Data(type=w128, Variant=w129) -> (data=w127:T23, error out=w126:errorcluster)  [unwired: 1 in]
                      n83 = local write "C7NI6703"(w127) -> ()
                    }
                    frame "VTL" {
                      n84 = local read "VTL"() -> (w132:string[])
                      n85 = Variant To Data(type=w132, Variant=w133) -> (data=w131:string[], error out=w130:errorcluster)  [unwired: 1 in]
                      n86 = local write "VTL"(w131) -> ()
                    }
                    frame "VDM-S" {
                      n87 = local read "VDM-S"() -> (w136:T27)
                      n88 = Variant To Data(type=w136, Variant=w137) -> (data=w135:T27, error out=w134:errorcluster)  [unwired: 1 in]
                      n89 = local write "VDM-S"(w135) -> ()
                    }
                    frame "C9NI6703" {
                      n90 = local read "C9NI6703"() -> (w140:T25)
                      n91 = Variant To Data(type=w140, Variant=w141) -> (data=w139:T25, error out=w138:errorcluster)  [unwired: 1 in]
                      n92 = local write "C9NI6703"(w139) -> ()
                    }
                    frame "C4_OUT_DIO96" {
                      n93 = local read "C4_OUT_DIO96"() -> (w144:T19)
                      n94 = Variant To Data(type=w144, Variant=w145) -> (data=w143:T19, error out=w142:errorcluster)  [unwired: 1 in]
                      n95 = local write "C4_OUT_DIO96"(w143) -> ()
                    }
                    frame "C1NI6071E" {
                      n96 = local read "C1NI6071E"() -> (w148:T14)
                      n97 = Variant To Data(type=w148, Variant=w149) -> (data=w147:T14, error out=w146:errorcluster)  [unwired: 1 in]
                      n98 = local write "C1NI6071E"(w147) -> ()
                    }
                  }
                  n99 = Unbundle By Name(w34) -> ("status"=w35:bool)  [unwired: 1 out]
                  n100 = case shown="True" w35 {
                    tunnel: w34 -> [w38 _]
                    tunnel: [w38 w39] -> w32
                    tunnel: w34 -> [_ w41]
                    tunnel: w33 -> [_ w40]
                    frame False {
                    }
                    frame True {
                      n101 = Bundle By Name(cluster=w41, "source"=w40) -> (w39:errorcluster)
                    }
                  }
                }
                n102 = Merge Errors(w29) -> (w28:errorcluster)
                n103 = case shown="Error .." w28 {
                  selector: w28 -> [_ w31]
                  frame No Error {
                  }
                  frame Error {
                    n104 = local write "error out"(w31) -> ()
                  }
                }
              }
            }
          }
          frame #1 {
            n105 = flat-sequence {
              tunnel: w152 -> [w156]
              tunnel: w151 -> [w155]
              tunnel: [w154] -> w150
              frame #0 {
                n106 = local read "C1NI6071E"() -> (w159:T14)
                n107 = local read "C2NI6071E"() -> (w158:T15)
                n108 = local read "C9NI6703"() -> (w157:T25)
                n109 = call "time-archive.vi"() -> ("output cluster"=w170:T1)
                n110 = local read "C2NI6071E"() -> (w171:T15)
                n111 = local read "C5_IN_DIO96"() -> (w165:T20)
                n112 = call "HT-HF-archive.vi"("C9NI6703"=w157, "C2NI6071E"=w158, "C1NI6071E"=w159, "archive in"=w170) -> ("archive out"=w172:T1)
                n113 = local read "VAM-A"() -> (w168:T30)
                n114 = local read "C1011NI6602"() -> (w166:T26)
                n115 = call "modulator.vi"("C2NI6071E"=w171, "archive in"=w172) -> ("archive out"=w169:T1)
                n116 = call "VAM-A-archive.vi"("VAM-A"=w168, "C5_IN_DIO96"=w165, "archive in"=w169) -> ("archive out"=w167:T1)
                n117 = call "sync-archive.vi"("C1011NI6602"=w166, "archive in"=w167) -> ("archive out"=w164:T1)
                n118 = local read "C6NI6703"() -> (w162:T22)
                n119 = local read "C7NI6703"() -> (w161:T23)
                n120 = local read "C8NI6703"() -> (w160:T24)
                n121 = call "water-archive.vi"("C1NI6071E"=w159, "archive in"=w164) -> ("archive out"=w163:T1)
                n122 = call "magnets-archive.vi"("archive in"=w163, "C6NI6703"=w162, "C7NI6703"=w161, "C8NI6703"=w160, "C1NI6071E"=w159) -> ("archive out"=w154:T1)
                "archive" <- w154
                n123 = call "tango_labview.vi"("previous"=w155, "i"=w156, "archive"=w154) -> ("error out"=w153:errorcluster)  [unwired: 8 in]
                n124 = local write "error out"(w153) -> ()
              }
            }
          }
        }
      }
    }
    frame #3 {
      n125 = flat-sequence {
        tunnel: w173 -> [w174]
        frame #0 {
          n126 = for {
            tunnel: w174 -> [w178] mode=indexing
            tunnel: [w177] -> w176 mode=indexing
            n127 = Close Variable Connection(11:w178) -> (0:w177:errorcluster)  [unwired: 1 in]
          }
          n128 = Merge Errors(w176) -> (w175:errorcluster)
          n129 = local write "error out"(w175) -> ()
        }
      }
    }
  }
